vi "dI-dV(V)_two devices_MFLI_MF-MD_K3636B_PK_V4.0.vi"() -> ()   [LabVIEW 2016]
uses:
  <instrlib>/Keithley 2600 Series/Public/Configure/Source/Configure Source (Limit).vi
  <instrlib>/Keithley 2600 Series/Public/Configure/Source/Configure Source (Range).vi
  <instrlib>/Zurich Instruments LabOne/Public/Configure/ziSetValueDouble.vi
  <instrlib>/Zurich Instruments LabOne/Public/Configure/ziGetValueDemodSampleEx.vi
  <instrlib>/Zurich Instruments LabOne/Zurich Instruments LabOne.lvlib
  <instrlib>/Keithley 2600 Series/Keithley 2600 Series.lvlib
panel:
  in  "MFLI autorange":bool
  in  "MFLI autophase":bool=TRUE
  out "data 2":dbl[](array[numeric])=[4987.521, -0.0022013766920000004, 3.480726954118042e-11, 5.034309826469514e-06, 6.914010210132466e-06, -1.6999999999999718, -8.499999999999859e-08]
  in  "Tab Control":enum32{"Device 1", "Device 2"}(tab)
  out "dI/dV vs DC Bias (Device 1)":cluster{dbl, "Field Reading":dbl}[](graph)=[{0.0014399891434999999, "Field Reading"=3.539984741655203e-05}, {0.0015442875115, "Field Reading"=3.479350977367112e-05}, {0.0015470007610000002, "Field Reading"=3.023097158131358e-05}, {0.00154666596, "Field Reading"=2.8749503676306814e-05}, {0.0015427451470000002, "Field Reading"=3.1774133983659106e-05}, {0.001535730355, "Field Reading"=3.5727767936050286e-05}, {0.001534129679, "Field Reading"=3.5111822569235866e-05}, {0.0015285104130000002, "Field Reading"=2.941147033935653e-05}, {0.0015257152995, "Field Reading"=2.9865278120159806e-05}, {0.0015236269315000001, "Field Reading"=3.240454202938594e-05}, {0.0015206740594999998, "Field Reading"=3.325907996536474e-05}, {0.0015153374560000004, "Field Reading"=3.1387152081909155e-05}, {0.001509890312, "Field Reading"=2.996223500052808e-05}, {0.0015049572590000002, "Field Reading"=3.099093031549478e-05}, {0.0015046650365000002, "Field Reading"=3.2089661815348154e-05}, {0.0015006593160000004, "Field Reading"=3.401106812223111e-05}, {0.001496798368, "Field Reading"=3.072884553542488e-05}, {0.001492131612, "Field Reading"=2.9522459100156508e-05}, {0.001486837714, "Field Reading"=3.153606057559728e-05}, {0.001484281524, "Field Reading"=3.175161419362383e-05}, {0.0014819942635, "Field Reading"=3.1800258559693947e-05}, {0.001478613938, "Field Reading"=3.126830433448307e-05}, {0.001469819908, "Field Reading"=2.7391136145857723e-05}, {0.0014674311730000001, "Field Reading"=2.8763716237227997e-05}, {0.001466370573, "Field Reading"=3.1089573912688234e-05}, {0.001461121836, "Field Reading"=3.307180706002982e-05}, {0.001458794033, "Field Reading"=3.121787322651838e-05}, {0.0014529708325000002, "Field Reading"=2.8244891952200815e-05}, {0.0014474971195, "Field Reading"=2.825445502582387e-05}, {0.0014433356870000003, "Field Reading"=3.072241009524203e-05}, {0.001438264611, "Field Reading"=2.995842383800983e-05}, {0.001435399206, "Field Reading"=3.3231202804746765e-05}, {0.0014323585335, "Field Reading"=3.1872234223847094e-05}, {0.0014242775069999998, "Field Reading"=3.0354032499741767e-05}, {0.0014239959914999999, "Field Reading"=3.237759520768794e-05}, {0.0014193896074999998, "Field Reading"=3.0402839737892528e-05}, {0.0014128105435000002, "Field Reading"=2.9377356291311724e-05}, {0.0014078315605000002, "Field Reading"=2.7797475631119178e-05}, {0.0014048058534999997, "Field Reading"=3.220364336714182e-05}, {0.001402497608, "Field Reading"=2.965534195305068e-05}, {0.0013961798765, "Field Reading"=3.067447845354369e-05}, {0.001390925393, "Field Reading"=3.11703676364192e-05}, {0.0013872433314999998, "Field Reading"=2.9243257786824305e-05}, {0.0013821559399999999, "Field Reading"=2.7398973790428333e-05}, {0.001377423483, "Field Reading"=3.008617236104539e-05}, {0.0013727005385, "Field Reading"=2.8406131733354052e-05}, {0.0013678423729999998, "Field Reading"=3.104440370058421e-05}, {0.0013666582235, "Field Reading"=3.047636089229375e-05}, {0.0013646590885000001, "Field Reading"=3.0184765629058295e-05}, {0.0013589371445, "Field Reading"=3.0307666179171986e-05}, {0.0013560817375000002, "Field Reading"=2.9523004632232655e-05}, {0.0013515789905000001, "Field Reading"=3.082554161062039e-05}, {0.0013447046144999999, "Field Reading"=3.106728717375647e-05}, {0.0013385220485, "Field Reading"=2.974868707473485e-05}, {0.0013374483420000003, "Field Reading"=2.8651427002743325e-05}, {0.0013321132029999998, "Field Reading"=3.055303541114044e-05}, {0.0013274556029999997, "Field Reading"=3.0637799613688364e-05}, {0.001321575341, "Field Reading"=3.1304129713072345e-05}, {0.0013141655734999998, "Field Reading"=2.7826668858596676e-05}, {0.0013122313234999999, "Field Reading"=2.938837368452147e-05}, {0.001307794673, "Field Reading"=3.2897151730779044e-05}, {0.0013034739785, "Field Reading"=3.0675530645251095e-05}, {0.001297746598, "Field Reading"=3.097612663835991e-05}, {0.0012949037034999998, "Field Reading"=3.226733852363065e-05}, {0.0012919954510000001, "Field Reading"=2.905384119263297e-05}, {0.0012888060755, "Field Reading"=2.9760444377154905e-05}, {0.0012821942274999997, "Field Reading"=3.152958550570822e-05}, {0.00127900604, "Field Reading"=2.9754485932266634e-05}, {0.0012753080475000002, "Field Reading"=2.7941981758265642e-05}, {0.001271380758, "Field Reading"=2.897923489602027e-05}, {0.0012681222019999998, "Field Reading"=3.0145087015586976e-05}, {0.0012625594059999998, "Field Reading"=2.9888548610541235e-05}, {0.0012601185500000001, "Field Reading"=2.892551585933325e-05}, {0.0012563334949999999, "Field Reading"=2.914199842671685e-05}, {0.0012516522169999998, "Field Reading"=3.106836766844688e-05}, {0.0012466661809999997, "Field Reading"=2.931506336795828e-05}, {0.0012434836825, "Field Reading"=3.012840945054606e-05}, {0.001238093922, "Field Reading"=3.013433569745804e-05}, {0.001232953168, "Field Reading"=2.8832248492968933e-05}, {0.0012277401725000003, "Field Reading"=2.8988694843593325e-05}, {0.0012234111989999998, "Field Reading"=3.0242812296195605e-05}, {0.0012216526839999998, "Field Reading"=3.089554375166708e-05}, {0.0012165614215, "Field Reading"=2.8698972585958197e-05}, {0.0012121334570000001, "Field Reading"=2.8319095802121462e-05}, {0.0012098926105, "Field Reading"=2.763785246347619e-05}, {0.0012050341640000002, "Field Reading"=2.973094124014038e-05}, {0.0012014678839999998, "Field Reading"=3.119323554533092e-05}, {0.00119644038, "Field Reading"=2.898124104108434e-05}, {0.001191083737, "Field Reading"=2.820127031302108e-05}, {0.0011860875315, "Field Reading"=2.798966210613631e-05}, {0.001181310497, "Field Reading"=3.053637390193424e-05}, {0.0011761192575000003, "Field Reading"=2.81047730972618e-05}, {0.001171179016, "Field Reading"=2.9913610446049883e-05}, {0.001166600119, "Field Reading"=2.9097237815217114e-05}, {0.0011662118055, "Field Reading"=2.9262892022534514e-05}, {0.0011637166605, "Field Reading"=2.7160091515073227e-05}, {0.0011595062940000002, "Field Reading"=2.7876172605800874e-05}, {0.0011525607660000004, "Field Reading"=2.9328265579124486e-05}, {0.0011474100155, "Field Reading"=2.780060002119802e-05}, {0.0011431688820000001, "Field Reading"=2.869299201580142e-05}, {0.0011373234735, "Field Reading"=2.9999385402787912e-05}, {0.0011332899885000002, "Field Reading"=2.7787092135107974e-05}, {0.0011274989709999998, "Field Reading"=2.832686477947079e-05}, {0.001121785455, "Field Reading"=2.877980796483004e-05}, {0.00111626547, "Field Reading"=2.9505815517494233e-05}, {0.0011128954825, "Field Reading"=2.6724980409852468e-05}, {0.001108690413, "Field Reading"=2.949081340220257e-05}, {0.0011035870930000001, "Field Reading"=2.893692751618776e-05}, {0.0010992904555, "Field Reading"=2.8973874312015976e-05}, {0.0010952211570000002, "Field Reading"=2.7947861861950238e-05}, {0.0010945930425, "Field Reading"=2.679006764938657e-05}, {0.001090257549, "Field Reading"=2.941158012860888e-05}, {0.0010852873185000001, "Field Reading"=2.865060713681523e-05}, {0.0010813640165000002, "Field Reading"=2.847363898604231e-05}, {0.0010766837349999998, "Field Reading"=2.7137000104643942e-05}, {0.0010729132935, "Field Reading"=2.7304465600784156e-05}, {0.001065158915, "Field Reading"=2.9474555033440265e-05}, {0.0010584838075000003, "Field Reading"=2.8951717323060825e-05}, {0.001055930303, "Field Reading"=2.8197744534596472e-05}, {0.001051506708, "Field Reading"=2.813935590078248e-05}, {0.001048655317, "Field Reading"=2.7457099511248944e-05}, {0.0010452859699999998, "Field Reading"=2.8129650859824848e-05}, {0.0010392103565000001, "Field Reading"=2.8386664538660484e-05}, {0.0010361408315, "Field Reading"=2.9145292073684028e-05}, {0.0010294199855, "Field Reading"=2.69594894037016e-05}, {0.001023745664, "Field Reading"=2.8633350551353477e-05}, {0.0010203086779999998, "Field Reading"=2.849731787795889e-05}, {0.0010141151010000004, "Field Reading"=2.83146550303579e-05}, {0.001008619177, "Field Reading"=2.773198825459167e-05}, {0.001002912347, "Field Reading"=2.725891765436985e-05}, {0.0009962556867, "Field Reading"=2.872385890178788e-05}, {0.00099223266475, "Field Reading"=2.708421117774275e-05}, {0.0009906227914999997, "Field Reading"=2.8873027104615078e-05}, {0.0009858544061999998, "Field Reading"=2.823219667588614e-05}, {0.00098009373775, "Field Reading"=2.775224423256098e-05}, {0.0009751813368, "Field Reading"=2.7704772924742456e-05}, {0.0009701312228999998, "Field Reading"=2.873380694247318e-05}, {0.0009644217738, "Field Reading"=2.6861226192122225e-05}, {0.0009578559449999998, "Field Reading"=2.85256105088142e-05}, {0.0009539425876000001, "Field Reading"=2.7924498092117206e-05}, {0.0009513818346500001, "Field Reading"=2.6099498824452862e-05}, {0.0009462421892499999, "Field Reading"=2.709904571514122e-05}, {0.0009418883127499999, "Field Reading"=2.768778165159705e-05}, {0.00093742923265, "Field Reading"=2.744018195436568e-05}, {0.0009327565449000002, "Field Reading"=2.6443486426550465e-05}, {0.0009290616069500001, "Field Reading"=2.7514798871704233e-05}, {0.00092673901585, "Field Reading"=2.794358683356436e-05}, {0.0009203088168000001, "Field Reading"=2.770115760603011e-05}, {0.0009145794246999999, "Field Reading"=2.7636471710395534e-05}, {0.00090842506875, "Field Reading"=2.6764078766304754e-05}, {0.00090077597955, "Field Reading"=2.7150526980398903e-05}, {0.00089646212625, "Field Reading"=2.7520786364024458e-05}, {0.0008906256886000002, "Field Reading"=2.7831637446333116e-05}, {0.0008856995292, "Field Reading"=2.631326422089245e-05}, {0.0008836259033, "Field Reading"=2.8233537331017953e-05}, {0.0008791930340999999, "Field Reading"=2.706401776615399e-05}, {0.00087525207395, "Field Reading"=2.7520214395887868e-05}, {0.0008724134060500001, "Field Reading"=2.8272804485753116e-05}, {0.0008646784291999998, "Field Reading"=2.731466430586837e-05}, {0.0008590569936000001, "Field Reading"=2.644908415508535e-05}, {0.0008540370289, "Field Reading"=2.652451844467208e-05}, {0.0008494558809500001, "Field Reading"=2.653246513039182e-05}, {0.0008430573263999999, "Field Reading"=2.717732781056327e-05}, {0.0008384341093, "Field Reading"=2.6343442524410912e-05}, {0.0008339046709999999, "Field Reading"=2.7015478964114357e-05}, {0.0008288371037499999, "Field Reading"=2.683564270016631e-05}, {0.0008243482518, "Field Reading"=2.7061071714567523e-05}, {0.0008224905806500001, "Field Reading"=2.7833471132280706e-05}, {0.0008167230211, "Field Reading"=2.7130822144725484e-05}, {0.0008139826599, "Field Reading"=2.7002573082600767e-05}, {0.00081011256475, "Field Reading"=2.6699793633173424e-05}, {0.00080354357335, "Field Reading"=2.6601707234183626e-05}, {0.0007998235963500002, "Field Reading"=2.7518846084862328e-05}, {0.00079305690065, "Field Reading"=2.5933886336674594e-05}, {0.0007881982002, "Field Reading"=2.628432329552786e-05}, {0.0007849861712, "Field Reading"=2.731155419644831e-05}, {0.00077924129495, "Field Reading"=2.6498316239054298e-05}, {0.00077386634115, "Field Reading"=2.661237385473222e-05}, {0.000772586717, "Field Reading"=2.683367763980429e-05}, {0.00076715324385, "Field Reading"=2.7552914639933646e-05}, {0.00076283068005, "Field Reading"=2.529660873922404e-05}, {0.0007584143292500001, "Field Reading"=2.6813040060921684e-05}, {0.0007518176841999999, "Field Reading"=2.6098759138522866e-05}, {0.0007503320720500001, "Field Reading"=2.7584507574510233e-05}, {0.0007454194233999999, "Field Reading"=2.6381757940346435e-05}, {0.0007392297915499999, "Field Reading"=2.6664197485017493e-05}, {0.0007335713615, "Field Reading"=2.5833327337248065e-05}, {0.0007310102463, "Field Reading"=2.6845579698123368e-05}, {0.0007250234232999999, "Field Reading"=2.5419589094556693e-05}, {0.0007188638338, "Field Reading"=2.664214168588533e-05}, {0.0007165599543499999, "Field Reading"=2.5592852741351857e-05}, {0.0007119381531, "Field Reading"=2.6259267949927292e-05}, {0.0007098633958499999, "Field Reading"=2.673315141982664e-05}, {0.0007047486914500001, "Field Reading"=2.6457039708447496e-05}, {0.0007025036933500001, "Field Reading"=2.5257856553764385e-05}, {0.0006956025043, "Field Reading"=2.628501082062639e-05}, {0.0006888174652, "Field Reading"=2.6144779354954198e-05}, {0.00068248965275, "Field Reading"=2.59082571996256e-05}, {0.0006772642433000001, "Field Reading"=2.5689649875885376e-05}, {0.0006708514852, "Field Reading"=2.6521326635999304e-05}, {0.0006693603533000001, "Field Reading"=2.548743026040851e-05}, {0.00066562013705, "Field Reading"=2.5431203693357216e-05}, {0.0006597756623499999, "Field Reading"=2.500251770448019e-05}, {0.0006545812863499999, "Field Reading"=2.5962650488942607e-05}, {0.00064974467235, "Field Reading"=2.5816920621354972e-05}, {0.0006442822826, "Field Reading"=2.5159993064492232e-05}, {0.0006390915108499999, "Field Reading"=2.660956856843091e-05}, {0.0006341380824, "Field Reading"=2.4788097750258985e-05}, {0.00062805348185, "Field Reading"=2.5239440389139205e-05}, {0.00062110338895, "Field Reading"=2.4843288989688017e-05}, {0.0006170477987, "Field Reading"=2.5471157379008036e-05}, {0.00061183636825, "Field Reading"=2.5198329240766945e-05}, {0.00060867340895, "Field Reading"=2.5026640430883117e-05}, {0.0006043969231999999, "Field Reading"=2.4532829122884805e-05}, {0.00059734108645, "Field Reading"=2.548186660127621e-05}, {0.0005915697426, "Field Reading"=2.53532964278651e-05}, {0.0005844833989, "Field Reading"=2.423295748808172e-05}, {0.0005813260316, "Field Reading"=2.530045533051123e-05}, {0.0005753792359999999, "Field Reading"=2.460499357020733e-05}, {0.00056967967195, "Field Reading"=2.476774868624248e-05}, {0.0005661936702499998, "Field Reading"=2.509068143160599e-05}, {0.0005608593239499999, "Field Reading"=2.508099804473662e-05}, {0.0005529609736, "Field Reading"=2.434759142994004e-05}, {0.0005465511633000001, "Field Reading"=2.472033680947642e-05}, {0.0005420742435999999, "Field Reading"=2.5294665456280207e-05}, {0.0005380521151000001, "Field Reading"=2.4446332182633667e-05}, {0.00053460002175, "Field Reading"=2.5219944239969312e-05}, {0.0005282012281499999, "Field Reading"=2.4927595151619875e-05}, {0.0005243503773499999, "Field Reading"=2.429086406589632e-05}, {0.000520241094, "Field Reading"=2.447064522503621e-05}, {0.0005154410257000001, "Field Reading"=2.4998108009755677e-05}, {0.0005086838760999998, "Field Reading"=2.4879104926386617e-05}, {0.0005030509692, "Field Reading"=2.52088880671345e-05}, {0.00049863510835, "Field Reading"=2.4460419844711307e-05}, {0.00049550265335, "Field Reading"=2.4131581166292184e-05}, {0.0004905697873499999, "Field Reading"=2.494270174489369e-05}, {0.00048358716750000004, "Field Reading"=2.4212429855592305e-05}, {0.00047998159185, "Field Reading"=2.456164211241159e-05}, {0.00047376262365, "Field Reading"=2.4452567434274788e-05}, {0.00046960355054999987, "Field Reading"=2.412365841886655e-05}, {0.00046395107535, "Field Reading"=2.468534893656029e-05}, {0.00045919463465, "Field Reading"=2.4664106355610692e-05}, {0.0004560322024, "Field Reading"=2.4709306593844774e-05}, {0.00045091883165, "Field Reading"=2.5036193006732655e-05}, {0.00044793911940000004, "Field Reading"=2.4227487109089688e-05}, {0.00044306784715, "Field Reading"=2.517362154516144e-05}, {0.0004394137854, "Field Reading"=2.4822170605215546e-05}, {0.0004343439982, "Field Reading"=2.4826098311102026e-05}, {0.00043020854309999993, "Field Reading"=2.4365481177436e-05}, {0.00042386048834999995, "Field Reading"=2.4189633858249927e-05}, {0.0004200018422500001, "Field Reading"=2.493572935828982e-05}, {0.00041879972499999995, "Field Reading"=2.5612108271423455e-05}, {0.0004126587697999999, "Field Reading"=2.4877559496683757e-05}, {0.00040355976715, "Field Reading"=2.4722490914043894e-05}, {0.00039708264615, "Field Reading"=2.507577663272283e-05}, {0.0003926418904, "Field Reading"=2.4859213827902027e-05}, {0.00038827582905000003, "Field Reading"=2.484408253104443e-05}, {0.00038332477235000003, "Field Reading"=2.4704709168198052e-05}, {0.00037710729935000004, "Field Reading"=2.449886332521343e-05}, {0.00036955482050000005, "Field Reading"=2.492090369325475e-05}, {0.00036543200345000006, "Field Reading"=2.5169323793221225e-05}, {0.0003600878789, "Field Reading"=2.4800261123674807e-05}, {0.0003548235144, "Field Reading"=2.4379325397423533e-05}, {0.00035248225715, "Field Reading"=2.5072746136214913e-05}, {0.00034454190035000003, "Field Reading"=2.5456751026618948e-05}, {0.0003373547338, "Field Reading"=2.5193594542978225e-05}, {0.00033139157100000005, "Field Reading"=2.5051119772538443e-05}, {0.00032845802785000003, "Field Reading"=2.4595954455078518e-05}, {0.00031977012094999994, "Field Reading"=2.5555066907659082e-05}, {0.00031229189740000004, "Field Reading"=2.525033796639999e-05}, {0.0003070755153, "Field Reading"=2.4959636421672204e-05}, {0.00030173855935, "Field Reading"=2.511727230190406e-05}, {0.00029700412215000004, "Field Reading"=2.485646423766272e-05}, {0.00029108035300000004, "Field Reading"=2.5254110212854904e-05}, {0.00028656948975, "Field Reading"=2.522063844237432e-05}, {0.00028121404, "Field Reading"=2.556225551518139e-05}, {0.0002768915544, "Field Reading"=2.5348455473893375e-05}, {0.00027314623445, "Field Reading"=2.596928765567297e-05}, {0.0002686946441, "Field Reading"=2.5794692974694497e-05}, {0.00026405435680000003, "Field Reading"=2.543835530019002e-05}, {0.00025547767255, "Field Reading"=2.5967526298170223e-05}, {0.00025577685035000004, "Field Reading"=2.5919987667737076e-05}, {0.0002475684079, "Field Reading"=2.6727985706790567e-05}, {0.00024244191250000002, "Field Reading"=2.6286364593496668e-05}, {0.00023755152825, "Field Reading"=2.6064537241575083e-05}, {0.00023369517364999997, "Field Reading"=2.644985803858201e-05}, {0.00022849653985000003, "Field Reading"=2.6469041455970916e-05}, {0.00022485788605, "Field Reading"=2.6674888198321487e-05}, {0.00021704982410000002, "Field Reading"=2.6884455180053248e-05}, {0.00021395987409999996, "Field Reading"=2.6883046699655776e-05}, {0.00020615774949999998, "Field Reading"=2.691626478195444e-05}, {0.00019933952025000002, "Field Reading"=2.7295263506282656e-05}, {0.00019463775365, "Field Reading"=2.737091952442337e-05}, {0.0001917452195, "Field Reading"=2.750745359434406e-05}, {0.00018569049294999999, "Field Reading"=2.8296354710335358e-05}, {0.0001812998034, "Field Reading"=2.8517056990434556e-05}, {0.00017823559865000002, "Field Reading"=2.8593356237518392e-05}, {0.0001737937612, "Field Reading"=2.861871554641695e-05}, {0.0001700427832, "Field Reading"=2.882651694872817e-05}, {0.00016924993275000002, "Field Reading"=2.9231417800203077e-05}, {0.00016525125185, "Field Reading"=2.9408133529936847e-05}, {0.00016064549415, "Field Reading"=2.9491500714110673e-05}, {0.00015722823585, "Field Reading"=3.06834394085974e-05}, {0.00015247696070000002, "Field Reading"=3.1570866964132345e-05}, {0.00014844088830000003, "Field Reading"=3.0781559929643716e-05}, {0.00014316816515, "Field Reading"=3.1728014939431126e-05}, {0.00013987931785, "Field Reading"=3.2125458999320914e-05}, {0.00013671200479999999, "Field Reading"=3.284340832072761e-05}, {0.0001366118402, "Field Reading"=3.3356574795994144e-05}, {0.00013220151095, "Field Reading"=3.440093673855362e-05}, {0.00012683921535, "Field Reading"=3.527437392777797e-05}, {0.00012226255275, "Field Reading"=3.521770490817976e-05}, {0.00011886821990000002, "Field Reading"=3.7293066150943776e-05}, {0.00011505580454999999, "Field Reading"=3.7984175461221217e-05}, {0.00011490839619999998, "Field Reading"=3.876432629075614e-05}, {0.00011242408390000002, "Field Reading"=3.978183890147552e-05}, {0.00011095500830000001, "Field Reading"=4.088599194523828e-05}, {0.00010964993754999999, "Field Reading"=4.234633944029058e-05}, {0.00010712797994999999, "Field Reading"=4.323003495776657e-05}, {0.00010219273870000001, "Field Reading"=4.3184482483381195e-05}, {9.631986105499999e-05, "Field Reading"=4.5991318352294254e-05}, {9.527548263e-05, "Field Reading"=4.7847802385840867e-05}, {9.252191591499999e-05, "Field Reading"=4.989054521708996e-05}, {8.8617183645e-05, "Field Reading"=5.046410957067126e-05}, {8.7566451025e-05, "Field Reading"=5.246608919854773e-05}, {8.3063985815e-05, "Field Reading"=5.321509081606504e-05}, {8.1176531035e-05, "Field Reading"=5.4582323046123394e-05}, {7.907132144500001e-05, "Field Reading"=5.5596712751055124e-05}, {7.827213049e-05, "Field Reading"=5.375508176128449e-05}, {7.841774079000001e-05, "Field Reading"=5.41199224112345e-05}, {7.4509621425e-05, "Field Reading"=5.2990999011949546e-05}, {7.320589597999999e-05, "Field Reading"=4.9695563411219837e-05}, {6.864829185e-05, "Field Reading"=4.520530671515756e-05}, {6.768719516000001e-05, "Field Reading"=4.0779634591056634e-05}, {6.4593064545e-05, "Field Reading"=3.5474813084590765e-05}, {6.2432785315e-05, "Field Reading"=3.084529558773287e-05}, {5.670509802000001e-05, "Field Reading"=2.4482478477827943e-05}, {5.3037691230000004e-05, "Field Reading"=1.773821775920651e-05}, {3.9517599785e-05, "Field Reading"=1.1809336674850649e-05}, {2.3342955355e-05, "Field Reading"=6.418252148735044e-06}, {-2.3944236415e-05, "Field Reading"=1.2874313254256006e-06}, {-0.00044288596725000005, "Field Reading"=1.7829705228301125e-06}, {-0.0005051536444, "Field Reading"=7.727922995125912e-06}, {-0.0005184544644500001, "Field Reading"=1.2556664668411418e-05}, {-0.0005268976066, "Field Reading"=1.8327868347778772e-05}, {-0.0005357643552, "Field Reading"=2.5035434821338e-05}, {-0.00053897130225, "Field Reading"=3.005580738892413e-05}, {-0.0005437766682, "Field Reading"=3.5395922163059525e-05}, {-0.00054553804945, "Field Reading"=4.150184448391502e-05}, {-0.0005511706686500001, "Field Reading"=4.6362694015758234e-05}, {-0.0005559163023499999, "Field Reading"=5.0130423425832106e-05}, {-0.0005543881889499999, "Field Reading"=5.335741502524605e-05}, {-0.0005592604063, "Field Reading"=5.411570066512388e-05}, {-0.0005605982064999999, "Field Reading"=5.465121419090429e-05}, {-0.0005629030597, "Field Reading"=5.475473056047824e-05}, {-0.0005643864397499999, "Field Reading"=5.501166190948225e-05}, {-0.0005697240176, "Field Reading"=5.31400833500483e-05}, {-0.0005718998929, "Field Reading"=5.319476368452034e-05}, {-0.0005761703489, "Field Reading"=5.0393322614515415e-05}, {-0.0005774828608, "Field Reading"=5.0117210546142615e-05}, {-0.0005792511608, "Field Reading"=4.763450052536487e-05}, {-0.00058427729175, "Field Reading"=4.6222596298617735e-05}, {-0.0005839630306500001, "Field Reading"=4.380763636273433e-05}, {-0.00058690824465, "Field Reading"=4.341709663323534e-05}, {-0.00058665562145, "Field Reading"=4.257979811006354e-05}, {-0.00059081148145, "Field Reading"=3.9733022729478504e-05}, {-0.0005917890384000001, "Field Reading"=3.922882008869421e-05}, {-0.0005928376371999999, "Field Reading"=3.872769287644023e-05}, {-0.0005963710346499999, "Field Reading"=3.786839615999292e-05}, {-0.00060304377145, "Field Reading"=3.614498242064283e-05}, {-0.00060705747125, "Field Reading"=3.5275522377934295e-05}, {-0.0006140201557499999, "Field Reading"=3.473781066261673e-05}, {-0.0006186047409, "Field Reading"=3.417365953948509e-05}, {-0.0006230151480999999, "Field Reading"=3.3079225624050956e-05}, {-0.0006267799413000001, "Field Reading"=3.251474967299545e-05}, {-0.00062886941835, "Field Reading"=3.2595210913017203e-05}, {-0.0006354146897, "Field Reading"=3.1488792156517215e-05}, {-0.0006380160867000001, "Field Reading"=3.120214389597704e-05}, {-0.00064386830235, "Field Reading"=3.125684953560282e-05}, {-0.0006480523066999999, "Field Reading"=3.0277268568468644e-05}, {-0.00064896883845, "Field Reading"=2.9768651422877856e-05}, {-0.00065340680835, "Field Reading"=2.960934130033152e-05}, {-0.00065811164405, "Field Reading"=2.9778240274563194e-05}, {-0.0006635885125500002, "Field Reading"=2.9376542680395736e-05}, {-0.00066648116515, "Field Reading"=2.852598488267133e-05}, {-0.0006695975924, "Field Reading"=2.7962131958752747e-05}, {-0.0006771186086500001, "Field Reading"=2.792167139815216e-05}, {-0.00067967447245, "Field Reading"=2.8593051848648095e-05}, {-0.0006853313692000001, "Field Reading"=2.827992652732514e-05}, {-0.00068965257765, "Field Reading"=2.733016829877469e-05}, {-0.00069658048195, "Field Reading"=2.718001106596477e-05}, {-0.00070006927375, "Field Reading"=2.697314805126955e-05}, {-0.0007063067703, "Field Reading"=2.7223623241350286e-05}, {-0.0007104617050500001, "Field Reading"=2.7221131662322604e-05}, {-0.0007158454615000001, "Field Reading"=2.6470268262583008e-05}, {-0.0007208107891, "Field Reading"=2.6360429428319376e-05}, {-0.00072542920115, "Field Reading"=2.6359508605806887e-05}, {-0.00073385787325, "Field Reading"=2.6465138066782306e-05}, {-0.0007344708868000001, "Field Reading"=2.5871440569675743e-05}, {-0.0007403752824, "Field Reading"=2.6927353113657345e-05}, {-0.0007431207725999999, "Field Reading"=2.5848786429398566e-05}, {-0.0007452998807500001, "Field Reading"=2.6119694708101804e-05}, {-0.0007487942998500001, "Field Reading"=2.636072535607038e-05}, {-0.0007553057972000001, "Field Reading"=2.6220748174400285e-05}, {-0.0007591562609500001, "Field Reading"=2.5886324889822564e-05}, {-0.0007657129732500001, "Field Reading"=2.553410085362131e-05}, {-0.0007685236647999999, "Field Reading"=2.5299635240635863e-05}, {-0.00077290691525, "Field Reading"=2.55529616681101e-05}, {-0.0007775658146, "Field Reading"=2.5593459123952253e-05}, {-0.00078298779045, "Field Reading"=2.5766911715028896e-05}, {-0.0007868718035000001, "Field Reading"=2.5329800845548382e-05}, {-0.00079214363745, "Field Reading"=2.5111997926056203e-05}, {-0.00079630611485, "Field Reading"=2.5219866414641062e-05}, {-0.0008009303386, "Field Reading"=2.576886341774044e-05}, {-0.0008081203436000001, "Field Reading"=2.5191674409460277e-05}, {-0.0008128989841, "Field Reading"=2.4659895923638357e-05}, {-0.00081992365215, "Field Reading"=2.557847433769245e-05}, {-0.0008227442695, "Field Reading"=2.491401355296153e-05}, {-0.0008269649726, "Field Reading"=2.494049970344901e-05}, {-0.0008320200444000001, "Field Reading"=2.498865870175516e-05}, {-0.0008362681799499999, "Field Reading"=2.507156110645498e-05}, {-0.00084043577685, "Field Reading"=2.4859819723508128e-05}, {-0.0008482895495, "Field Reading"=2.4756956203228876e-05}, {-0.0008519631337, "Field Reading"=2.514257946106073e-05}, {-0.00085482501865, "Field Reading"=2.5190629511597944e-05}, {-0.00086115240905, "Field Reading"=2.4968169535876815e-05}, {-0.0008669621674000001, "Field Reading"=2.46774175944596e-05}, {-0.0008739308819, "Field Reading"=2.4956204388644077e-05}, {-0.00087753713925, "Field Reading"=2.501595182353837e-05}, {-0.0008833726753999999, "Field Reading"=2.4753643027387e-05}, {-0.0008833791037499998, "Field Reading"=2.4572507911983235e-05}, {-0.0008900118714, "Field Reading"=2.452449557800081e-05}, {-0.0008975926323500002, "Field Reading"=2.5742257691681753e-05}, {-0.0009049993725499999, "Field Reading"=2.483570784067544e-05}, {-0.0009106274022499999, "Field Reading"=2.4632699872762128e-05}, {-0.0009144832965, "Field Reading"=2.500623968887879e-05}, {-0.0009195275330000001, "Field Reading"=2.4533211575573895e-05}, {-0.0009253394478499998, "Field Reading"=2.46566289914237e-05}, {-0.0009295518563999999, "Field Reading"=2.4711007529370937e-05}, {-0.0009339636874499998, "Field Reading"=2.494095987800124e-05}, {-0.0009419215269, "Field Reading"=2.488276682153817e-05}, {-0.0009440282936000001, "Field Reading"=2.5362278074920992e-05}, {-0.0009520676295000001, "Field Reading"=2.4875495822276945e-05}, {-0.0009562295733499999, "Field Reading"=2.471985815352984e-05}, {-0.00096403001325, "Field Reading"=2.501400012487715e-05}, {-0.0009668210693999998, "Field Reading"=2.504545001027246e-05}, {-0.0009700857615000001, "Field Reading"=2.4825614172064623e-05}, {-0.0009741633754, "Field Reading"=2.508908994201125e-05}, {-0.0009786747900500002, "Field Reading"=2.547992134200255e-05}, {-0.0009831387377500001, "Field Reading"=2.4987278578304335e-05}, {-0.00098489078335, "Field Reading"=2.4799577546204462e-05}, {-0.00099149049345, "Field Reading"=2.517378273657648e-05}, {-0.0010008897577999999, "Field Reading"=2.501285906441021e-05}, {-0.0010047693850000002, "Field Reading"=2.517146386711981e-05}, {-0.001010887702, "Field Reading"=2.474528686486035e-05}, {-0.0010154381795, "Field Reading"=2.517950175218433e-05}, {-0.0010194920305, "Field Reading"=2.4943020751004832e-05}, {-0.001025390771, "Field Reading"=2.5059853035305155e-05}, {-0.0010319175369999998, "Field Reading"=2.5111712727938145e-05}, {-0.0010339942155000001, "Field Reading"=2.4965884900478457e-05}, {-0.0010387866259999998, "Field Reading"=2.4624146165130197e-05}, {-0.0010432882684999999, "Field Reading"=2.4974885798460943e-05}, {-0.001050285043, "Field Reading"=2.549970160202571e-05}, {-0.0010532131215, "Field Reading"=2.509936185921828e-05}, {-0.0010605935165, "Field Reading"=2.4679251006447366e-05}, {-0.0010649837745, "Field Reading"=2.534172622465245e-05}, {-0.0010699723350000002, "Field Reading"=2.5117530228594704e-05}, {-0.0010740878005, "Field Reading"=2.550911754774814e-05}, {-0.0010803877715, "Field Reading"=2.5590996285863874e-05}, {-0.0010843786035, "Field Reading"=2.532765980863689e-05}, {-0.0010869649905000003, "Field Reading"=2.504883136678769e-05}, {-0.0010908974514999999, "Field Reading"=2.5356105465320954e-05}, {-0.0010965432235000001, "Field Reading"=2.619328160076385e-05}, {-0.0011007961549999998, "Field Reading"=2.5554603625258115e-05}, {-0.0011068035015, "Field Reading"=2.486060925242396e-05}, {-0.0011102547485, "Field Reading"=2.5991799787265172e-05}, {-0.001114113474, "Field Reading"=2.5382768369364457e-05}, {-0.001120774231, "Field Reading"=2.560148212416169e-05}, {-0.0011256925015, "Field Reading"=2.535548059743797e-05}, {-0.0011314602925, "Field Reading"=2.4739011324466265e-05}, {-0.001133669728, "Field Reading"=2.4926499499317303e-05}, {-0.0011401122615000002, "Field Reading"=2.6136534239552487e-05}, {-0.0011450076414999998, "Field Reading"=2.5417209022334496e-05}, {-0.0011529607145000001, "Field Reading"=2.5698245491377132e-05}, {-0.0011577730315, "Field Reading"=2.6174948723676456e-05}, {-0.0011613708525, "Field Reading"=2.659495330024166e-05}, {-0.0011653017159999998, "Field Reading"=2.636519742423141e-05}, {-0.0011721344295000003, "Field Reading"=2.570186047778655e-05}, {-0.0011761560885000001, "Field Reading"=2.580018779418553e-05}, {-0.0011814869265000002, "Field Reading"=2.679967128975373e-05}, {-0.0011864733475, "Field Reading"=2.6239134735091276e-05}, {-0.0011893287184999999, "Field Reading"=2.5374579332499126e-05}, {-0.0011953142824999998, "Field Reading"=2.5780689417062888e-05}, {-0.0011998791505, "Field Reading"=2.6470977603648504e-05}, {-0.0012066721364999999, "Field Reading"=2.664068368641496e-05}, {-0.0012114344315000002, "Field Reading"=2.632872486761017e-05}, {-0.0012160587375, "Field Reading"=2.5944407033586477e-05}, {-0.0012206377089999999, "Field Reading"=2.6334788208618243e-05}, {-0.0012236480440000002, "Field Reading"=2.670412347473009e-05}, {-0.0012285901605, "Field Reading"=2.6385921389739756e-05}, {-0.0012339220824999998, "Field Reading"=2.6999631404588567e-05}, {-0.0012376608755, "Field Reading"=2.6434169175038227e-05}, {-0.0012383639600000002, "Field Reading"=2.7166475988494615e-05}, {-0.001244508114, "Field Reading"=2.7006307012055734e-05}, {-0.0012503813314999998, "Field Reading"=2.6804753979359723e-05}, {-0.0012582029339999999, "Field Reading"=2.7125886090709387e-05}, {-0.0012611768514999998, "Field Reading"=2.6236926946293805e-05}, {-0.0012639195255000001, "Field Reading"=2.6782100715955357e-05}, {-0.0012664462864999998, "Field Reading"=2.6554221045846453e-05}, {-0.0012745661625000002, "Field Reading"=2.6738797232680578e-05}, {-0.0012795817480000002, "Field Reading"=2.612651037782988e-05}, {-0.001282848078, "Field Reading"=2.6570038951477157e-05}, {-0.0012915996034999998, "Field Reading"=2.6500769220546404e-05}, {-0.0012962128675, "Field Reading"=2.6356774643710844e-05}, {-0.0013026879300000003, "Field Reading"=2.6794012485918364e-05}, {-0.001306773918, "Field Reading"=2.7001691426995927e-05}, {-0.0013085944285, "Field Reading"=2.6839401737944833e-05}, {-0.0013154063285, "Field Reading"=2.75133916908824e-05}, {-0.0013198725589999996, "Field Reading"=2.6462978869963258e-05}, {-0.0013259697260000001, "Field Reading"=2.7091350944690248e-05}, {-0.0013300431595, "Field Reading"=2.684988080475616e-05}, {-0.0013364990009999997, "Field Reading"=2.6864969015282564e-05}, {-0.001340103434, "Field Reading"=2.7074621441558483e-05}, {-0.0013446258885, "Field Reading"=2.658828009406131e-05}, {-0.0013491423099999999, "Field Reading"=2.6963634968708878e-05}, {-0.0013542443670000002, "Field Reading"=2.691242477475801e-05}, {-0.0013551154554999997, "Field Reading"=2.7408320729240955e-05}, {-0.0013603372705, "Field Reading"=2.6575551393078534e-05}, {-0.0013646557795, "Field Reading"=2.7190974281437918e-05}, {-0.0013668146055000004, "Field Reading"=2.7091075111983577e-05}, {-0.001374753727, "Field Reading"=2.697325299903679e-05}, {-0.0013790293659999998, "Field Reading"=2.6961363555538916e-05}, {-0.00138246604, "Field Reading"=2.7520779720375435e-05}, {-0.0013878468099999999, "Field Reading"=2.718517663643333e-05}, {-0.0013928858559999998, "Field Reading"=2.7704228552271802e-05}, {-0.0014003405395000001, "Field Reading"=2.7411265301839192e-05}, {-0.0014052482485, "Field Reading"=2.670572063970964e-05}, {-0.0014094181559999998, "Field Reading"=2.726189036114562e-05}, {-0.0014162599145, "Field Reading"=2.681430077596952e-05}, {-0.0014206207965000001, "Field Reading"=2.7064647645767718e-05}, {-0.001422804084, "Field Reading"=2.8156356118263624e-05}, {-0.0014294806425000002, "Field Reading"=2.816675161874044e-05}, {-0.0014314233145, "Field Reading"=2.836763394568079e-05}, {-0.0014342185515, "Field Reading"=2.7308793127739642e-05}, {-0.001438674201, "Field Reading"=2.7657009178311895e-05}, {-0.0014409701235000001, "Field Reading"=2.7488171670496874e-05}, {-0.0014457268345, "Field Reading"=2.7798227130753798e-05}, {-0.0014498154880000001, "Field Reading"=2.8672170248405528e-05}, {-0.0014527951515000003, "Field Reading"=2.814285356967082e-05}, {-0.001459003039, "Field Reading"=2.82471579598307e-05}, {-0.0014630158200000002, "Field Reading"=2.8591425967924597e-05}, {-0.0014650744875, "Field Reading"=2.8631034080160183e-05}, {-0.0014712758715, "Field Reading"=2.668663665944264e-05}, {-0.0014757668640000001, "Field Reading"=2.8148492175449524e-05}, {-0.001482266591, "Field Reading"=2.763950928937077e-05}, {-0.0014872015745000002, "Field Reading"=2.8529012683654844e-05}, {-0.0014917270425, "Field Reading"=2.7165504576848428e-05}, {-0.0014975122574999997, "Field Reading"=2.9116578377773362e-05}, {-0.0015011177470000002, "Field Reading"=2.9099655059723038e-05}, {-0.0015038803205000002, "Field Reading"=2.8669345250550533e-05}, {-0.0015074313985, "Field Reading"=2.818280079714946e-05}, {-0.0015148559224999998, "Field Reading"=2.8215570568220332e-05}, {-0.001518905766, "Field Reading"=2.8610697108516978e-05}, {-0.0015222922020000002, "Field Reading"=2.9179363255422852e-05}, {-0.0015271702825, "Field Reading"=2.8297513239277402e-05}, {-0.0015295628110000002, "Field Reading"=2.6834126964094553e-05}, {-0.0015345809465, "Field Reading"=2.792914219067848e-05}, {-0.0015406848935000002, "Field Reading"=2.829254332544149e-05}, {-0.0015452536425, "Field Reading"=2.7468626467104844e-05}, {-0.0015502011235000001, "Field Reading"=2.8621735203641882e-05}, {-0.0015551437465, "Field Reading"=2.761130630469376e-05}, {-0.0015605372085, "Field Reading"=2.6936326850914844e-05}, {-0.00156492463, "Field Reading"=2.827693033016408e-05}, {-0.0015669900035, "Field Reading"=2.8411256496876676e-05}, {-0.001571965995, "Field Reading"=2.7943121786343522e-05}, {-0.0015753530605, "Field Reading"=2.8376384388796066e-05}, {-0.0015807512605, "Field Reading"=2.978102067631948e-05}, {-0.0015864854214999997, "Field Reading"=3.004064400789514e-05}, {-0.001591627528, "Field Reading"=2.8055249135705818e-05}, {-0.0015950191769999998, "Field Reading"=2.949038938594226e-05}, {-0.001598778914, "Field Reading"=2.9143754000256578e-05}, {-0.0016050448364999998, "Field Reading"=2.8098754487818475e-05}, {-0.001609540912, "Field Reading"=2.8442217210198144e-05}, {-0.0016140246455, "Field Reading"=2.985325361373035e-05}, {-0.0016178020025, "Field Reading"=2.8824802231216225e-05}, {-0.0016212227885, "Field Reading"=2.9469524633747556e-05}, {-0.0016286767495, "Field Reading"=2.9330753129539258e-05}, {-0.0016321227720000001, "Field Reading"=2.863090278005049e-05}, {-0.0016345999689999998, "Field Reading"=2.945281627501967e-05}, {-0.0016406766190000001, "Field Reading"=3.0509889915088457e-05}, {-0.0016433718110000003, "Field Reading"=2.8234805007257297e-05}, {-0.0016475666914999999, "Field Reading"=3.0100850627959698e-05}, {-0.0016489186579999998, "Field Reading"=2.9164854213138128e-05}, {-0.0016580827585, "Field Reading"=2.820079826409188e-05}, {-0.0016634588009999999, "Field Reading"=2.948371397680206e-05}, {-0.001666819524, "Field Reading"=3.158853041941357e-05}, {-0.0016682677344999996, "Field Reading"=2.9247798446691426e-05}, {-0.0016724487044999996, "Field Reading"=2.820867278535577e-05}, {-0.001675465457, "Field Reading"=2.9148426410644136e-05}, {-0.0016796926040000004, "Field Reading"=3.063202582139158e-05}, {-0.0016869314475000002, "Field Reading"=3.084701188943617e-05}, {-0.0016899639645000003, "Field Reading"=3.0370369902881822e-05}, {-0.0016937376340000001, "Field Reading"=2.7594955047741704e-05}, {-0.0016975268330000001, "Field Reading"=2.9553103747146036e-05}, {-0.0017007798195, "Field Reading"=3.098220513643231e-05}, {-0.0017058537240000002, "Field Reading"=3.148168938244963e-05}, {-0.0017080639914999998, "Field Reading"=2.9579034160154674e-05}, {-0.0017110607904999998, "Field Reading"=2.7611498995410022e-05}, {-0.00171618452, "Field Reading"=3.0474417966750653e-05}, {-0.0017202808825, "Field Reading"=3.070057693750096e-05}, {-0.001727383138, "Field Reading"=3.162016826431228e-05}, {-0.0017310668390000002, "Field Reading"=2.9615498667636423e-05}, {-0.0017346550049999999, "Field Reading"=2.7453062758722423e-05}, {-0.0017379636470000002, "Field Reading"=3.043968244331558e-05}, {-0.001743127447, "Field Reading"=3.17359438510126e-05}, {-0.0017448500155000002, "Field Reading"=2.839198714788124e-05}, {-0.0017493435330000005, "Field Reading"=2.9537518085808404e-05}, {-0.001755053409, "Field Reading"=3.0267484755413558e-05}, {-0.00176169259, "Field Reading"=2.898267506640183e-05}, {-0.001762598, "Field Reading"=3.0300716833725148e-05}, {-0.0017671871915000002, "Field Reading"=3.080667331394037e-05}, {-0.0017705653674999998, "Field Reading"=3.0361398500792185e-05}, {-0.0017746671585000002, "Field Reading"=3.1106312903425585e-05}, {-0.0017783549920000002, "Field Reading"=2.9862151905111414e-05}, {-0.0017815493589999998, "Field Reading"=2.8501485801207906e-05}, {-0.001785276159, "Field Reading"=3.076140660046423e-05}, {-0.0017922079725, "Field Reading"=2.9058295998685708e-05}, {-0.0017961523975, "Field Reading"=2.8734206677692602e-05}, {-0.001799212137, "Field Reading"=3.137923256237406e-05}, {-0.0018059357504999999, "Field Reading"=3.179509940643667e-05}, {-0.0018087371615, "Field Reading"=3.228147459514946e-05}, {-0.0018160808960000004, "Field Reading"=3.293210062424598e-05}, {-0.001820149226, "Field Reading"=2.9163517417526188e-05}, {-0.0018234938499999999, "Field Reading"=3.1017183743855944e-05}, {-0.0018273520249999999, "Field Reading"=3.221606893453561e-05}, {-0.0018319088200000003, "Field Reading"=3.192150001949322e-05}, {-0.0018365081444999998, "Field Reading"=2.9959217951422412e-05}, {-0.0018389348775000001, "Field Reading"=2.789130975261861e-05}, {-0.0018452034285000001, "Field Reading"=3.17080422471979e-05}, {-0.0018500183390000005, "Field Reading"=3.2394673320763635e-05}, {-0.0018521909855, "Field Reading"=2.965997929508729e-05}, {-0.0018548242490000002, "Field Reading"=3.097145110133598e-05}, {-0.001858377908, "Field Reading"=3.0337147697741198e-05}, {-0.0018604670740000003, "Field Reading"=3.1532452120555806e-05}, {-0.0018638291629999998, "Field Reading"=3.270858332747162e-05}, {-0.0018671888555, "Field Reading"=3.0894156475968046e-05}, {-0.0018717320815, "Field Reading"=2.845308959992079e-05}, {-0.0018754390465, "Field Reading"=3.060980262409263e-05}, {-0.00187866943, "Field Reading"=3.2072999511849786e-05}, {-0.0018851805094999997, "Field Reading"=3.2173443940677715e-05}, {-0.001889215759, "Field Reading"=2.7966094150345777e-05}, {-0.0018937420315000002, "Field Reading"=3.0311161349639648e-05}, {-0.001897686686, "Field Reading"=3.274133195580933e-05}, {-0.001903061709, "Field Reading"=3.4094299280965945e-05}, {-0.0019071081000000003, "Field Reading"=3.082707587247123e-05}, {-0.001909890899, "Field Reading"=2.9702084757446434e-05}, {-0.0019168490989999998, "Field Reading"=2.976508458726319e-05}, {-0.001920534376, "Field Reading"=3.2748509436225333e-05}, {-0.001924188862, "Field Reading"=3.094510845635821e-05}, {-0.0019281178400000001, "Field Reading"=2.9363437972452403e-05}, {-0.001935024801, "Field Reading"=2.965602205230533e-05}, {-0.0019368541310000001, "Field Reading"=3.349567018076371e-05}, {-0.0019395661065, "Field Reading"=3.11382374433274e-05}, {-0.0019443560055, "Field Reading"=3.272398904929557e-05}, {-0.0019478042074999996, "Field Reading"=2.9959093799175477e-05}, {-0.0019505890269999999, "Field Reading"=3.21476349140092e-05}, {-0.001955327842, "Field Reading"=3.481998753888036e-05}, {-0.001960148591, "Field Reading"=3.2242893449899114e-05}, {-0.0019617751235, "Field Reading"=2.8580219684115152e-05}, {-0.0019670099799999996, "Field Reading"=3.0965338889550495e-05}, {-0.001969988556, "Field Reading"=3.32122447642128e-05}, {-0.0019757059180000006, "Field Reading"=3.253687631425346e-05}, {-0.0019789746340000006, "Field Reading"=2.742705969097034e-05}, {-0.0019831723155000003, "Field Reading"=3.196348596581089e-05}, {-0.0019871198235000007, "Field Reading"=2.900741316885134e-05}, {-0.0019899086759999998, "Field Reading"=3.543967510024724e-05}, {-0.0019937853094999995, "Field Reading"=3.032039195721649e-05}, {-0.001997198822, "Field Reading"=3.124126865424502e-05}, {-0.002004981853, "Field Reading"=2.8959096894867582e-05}, {-0.0020066316215, "Field Reading"=2.738232973306536e-05}, {-0.0020110788365, "Field Reading"=3.162264271194698e-05}]
  out "DC Voltage (V)":dbl=-0.0020110788365
  out "dI (A)":dbl=8.848779425879616e-11
  out "dV (V)":dbl=2.798241597479316e-06
  out "dI/dV (ohm)":dbl=3.162264271194698e-05
  out "Vset (V)":dbl=-1.6999999999999718
  in  "Nanovoltmeter 2182A VISA (Device1)":refnum<visa-resource-name>="GPIB0::4::INSTR"
  in  "MFLI Device 1 Address\n(connected to Channel A of K2635B)":string="DEV4382"
  in  "File Name Device 1":string="005_MA2479_[Dev110]_40uV_50pA_17.7777Hz_4thorder_300ms_2T_measureX_float_20xaverage"
  in  "From 1":dbl[](array[numeric])=[1.645, 0.5, 0.025, -0.035, -0.54] min=-3000.0 max=3000.0 format="%.2e"
  in  "To 1":dbl[](array[numeric])=[0.5, 0.025, -0.035, -0.54, -1.65] min=-3000.0 max=3000.0 format="%.2e"
  in  "Step 1":dbl[](array[numeric])=[0.005, 0.002, 0.001, 0.002, 0.005] min=-3000.0 max=3000.0 format="%.1e"
  in  "Resistance used for DC (Device 1) (ohm)":dbl=40000000.0 format="%#_13g"
  in  "DC Voltage averaging (Device 1)":dbl=20.0 format="%#_13g"
  in  "MFLI Averaging (Device1)":dbl=20.0 format="%#_13g"
  in  "MFLI Device 1 Delay (s)":dbl=4.0
  in  "MFLI Device 2 Address\n(connected to Channel B of K2635B)":string="DEV4496"
  in  "Resistance used for DC (ohm) 2":dbl=20000000.0 format="%#_13g"
  in  "Nanovoltmeter 2182a VISA (Device 2)":refnum<visa-resource-name>="GPIB0::7::INSTR"
  in  "File Name Device 2":string="006_MA2479_[Dev90]_40uV_33pA_7.919Hz_4thorder_300ms_2T_measureX_float_20xaverage"
  in  "MFLI Device 2 Delay (s)":dbl=4.0
  in  "From 3":dbl[](array[numeric])=[1.65, 0.5, 0.025, -0.035, -0.54] min=-3000.0 max=3000.0 format="%.2e"
  in  "To 3":dbl[](array[numeric])=[0.5, 0.025, -0.035, -0.54, 1.65] min=-3000.0 max=3000.0 format="%.2e"
  in  "Step 3":dbl[](array[numeric])=[0.005, 0.002, 0.001, 0.002, 0.005] min=-3000.0 max=3000.0 format="%.1e"
  out "dI/dV vs DC Bias (Device 2)":cluster{dbl, "Field Reading":dbl}[](graph)=[{0.0016536990575000004, "Field Reading"=1.0549538115165888e-05}, {0.001778714152, "Field Reading"=1.2441234786608795e-05}, {0.0017803415199999998, "Field Reading"=2.288258346714741e-05}, {0.0017755957270000002, "Field Reading"=1.318154414138772e-05}, {0.0017698667430000002, "Field Reading"=6.944765527644103e-06}, {0.0017656221274999998, "Field Reading"=1.2547089254133368e-05}, {0.0017618064770000004, "Field Reading"=8.29737778524207e-06}, {0.0017527998860000006, "Field Reading"=1.1494966792116706e-05}, {0.0017486110414999998, "Field Reading"=1.0588496845450188e-05}, {0.0017437714000000004, "Field Reading"=1.1963581383580064e-05}, {0.0017407059809999997, "Field Reading"=5.731216326454031e-06}, {0.0017423811614999999, "Field Reading"=5.30625093465625e-06}, {0.0017370860829999998, "Field Reading"=1.128100400443151e-05}, {0.0017338522185, "Field Reading"=2.123556094372534e-05}, {0.0017289355484999998, "Field Reading"=1.117670770827346e-05}, {0.0017188669980000002, "Field Reading"=1.0835120440598476e-05}, {0.0017189288765000002, "Field Reading"=2.0192283145985024e-05}, {0.0017122291565000002, "Field Reading"=2.4785742477983657e-05}, {0.0017076021445, "Field Reading"=1.0589077020565965e-05}, {0.0017052432175, "Field Reading"=1.3759186431392488e-05}, {0.0017045775195000002, "Field Reading"=1.537687077784978e-05}, {0.0016996537305, "Field Reading"=1.1320197025124775e-05}, {0.0016953896885, "Field Reading"=4.111009127394301e-06}, {0.001693602352, "Field Reading"=7.2063798052163e-06}, {0.0016863126914999998, "Field Reading"=7.631719043699821e-06}, {0.0016810597275000003, "Field Reading"=1.242338892269991e-05}, {0.001677800643, "Field Reading"=1.3726170510015826e-05}, {0.0016768591975, "Field Reading"=1.0512885770990247e-05}, {0.0016675404135000002, "Field Reading"=4.75578215245112e-06}, {0.0016654858590000002, "Field Reading"=2.027029645969641e-05}, {0.0016586733520000002, "Field Reading"=1.281946079436041e-05}, {0.0016534433870000003, "Field Reading"=6.055607337868207e-06}, {0.0016497589909999998, "Field Reading"=1.3221236417835137e-05}, {0.001642726164, "Field Reading"=8.223559087892218e-06}, {0.001632876745, "Field Reading"=1.590634888399578e-05}, {0.0016237432070000002, "Field Reading"=9.173376660503408e-06}, {0.0016184162055, "Field Reading"=1.6312838752629565e-05}, {0.001618065896, "Field Reading"=2.3731068197859222e-05}, {0.001618770715, "Field Reading"=1.0331543245369263e-05}, {0.0016073995474999998, "Field Reading"=6.470124896934937e-06}, {0.0015978612295, "Field Reading"=1.600525933976539e-05}, {0.0015944400540000001, "Field Reading"=1.7397689972344422e-05}, {0.0015942704750000001, "Field Reading"=1.2432826943314632e-05}, {0.0015882790550000002, "Field Reading"=9.114399852548662e-06}, {0.0015826422325, "Field Reading"=9.258860509987068e-06}, {0.0015787430519999999, "Field Reading"=1.8612913508766953e-05}, {0.001574898086, "Field Reading"=1.3182472661864731e-05}, {0.0015700212479999999, "Field Reading"=1.7030521500463586e-05}, {0.0015719165115, "Field Reading"=1.3417541074045366e-05}, {0.0015680138215, "Field Reading"=9.850868553296031e-06}, {0.00156138302, "Field Reading"=1.2254888938026482e-05}, {0.0015595287044999997, "Field Reading"=2.0389817245679517e-05}, {0.0015526102765, "Field Reading"=7.176125737368203e-06}, {0.0015470934585, "Field Reading"=1.474392740423153e-05}, {0.0015406487560000002, "Field Reading"=6.692190816914176e-06}, {0.0015367547195000001, "Field Reading"=1.5447400080198977e-05}, {0.001535941625, "Field Reading"=6.532333325868927e-06}, {0.0015307425095000002, "Field Reading"=1.7413230844513688e-05}, {0.0015260549489999999, "Field Reading"=1.0434230642215218e-05}, {0.0015176100955, "Field Reading"=1.2101733376211772e-05}, {0.001511127055, "Field Reading"=1.0178996127798104e-05}, {0.001507063141, "Field Reading"=1.4738737572511442e-05}, {0.0015027795215, "Field Reading"=8.262259757536864e-06}, {0.0014955986639999998, "Field Reading"=1.6465762643777065e-05}, {0.001489394298, "Field Reading"=1.426412095304383e-05}, {0.0014849224090000002, "Field Reading"=4.5222377370536295e-06}, {0.0014789590254999999, "Field Reading"=1.752265421591796e-05}, {0.0014734957045, "Field Reading"=7.086367144957606e-06}, {0.0014665331415, "Field Reading"=1.8102862099937696e-05}, {0.0014644652449999998, "Field Reading"=7.316505619558816e-06}, {0.001459879062, "Field Reading"=1.37617730508661e-05}, {0.001456597234, "Field Reading"=7.997778680662308e-06}, {0.001455313604, "Field Reading"=1.9441226029715573e-05}, {0.0014529164155, "Field Reading"=1.0715716208961658e-05}, {0.0014459223660000001, "Field Reading"=1.0707737364503455e-05}, {0.001443026579, "Field Reading"=9.286061057576923e-06}, {0.0014390227154999998, "Field Reading"=1.7041859386511388e-05}, {0.001435458936, "Field Reading"=1.0920769827263233e-05}, {0.0014284858615, "Field Reading"=1.3097238678707195e-05}, {0.0014155124364999998, "Field Reading"=1.4943301047674539e-05}, {0.0014111933845, "Field Reading"=5.8346849278326184e-06}, {0.0014089356844999997, "Field Reading"=1.6267991558672235e-05}, {0.001400876774, "Field Reading"=6.2157367659959844e-06}, {0.0013967058315, "Field Reading"=1.4893518977580172e-05}, {0.0013969721584999998, "Field Reading"=6.624033742801718e-06}, {0.0013922511495, "Field Reading"=1.2408363902223439e-05}, {0.0013878740965000001, "Field Reading"=1.1728994786990398e-05}, {0.0013784779875, "Field Reading"=1.6012598335679754e-05}, {0.001373894446, "Field Reading"=1.1607856045479023e-05}, {0.001376841956, "Field Reading"=1.3706169986026481e-05}, {0.0013736510590000002, "Field Reading"=1.2806127733243977e-05}, {0.0013650868689999997, "Field Reading"=8.195390358346867e-06}, {0.0013547451064999999, "Field Reading"=1.6565652587357594e-05}, {0.0013496873084999999, "Field Reading"=8.17962273174124e-06}, {0.001344070701, "Field Reading"=1.598311850023392e-05}, {0.0013365678835, "Field Reading"=1.68947157592058e-05}, {0.0013371844205000002, "Field Reading"=6.9113858577387e-06}, {0.0013289714789999998, "Field Reading"=1.6095504394402362e-05}, {0.0013241351944999996, "Field Reading"=8.708982244850283e-06}, {0.0013160219430000003, "Field Reading"=1.4995882937862019e-05}, {0.0013141926445, "Field Reading"=7.715603867966122e-06}, {0.001307578675, "Field Reading"=1.0508798844202823e-05}, {0.0013072095634999998, "Field Reading"=1.0844911550062126e-05}, {0.0013007955015, "Field Reading"=1.27924273437336e-05}, {0.0012968136035, "Field Reading"=1.2856378064505285e-05}, {0.0012935500455000001, "Field Reading"=4.230795106372986e-06}, {0.0012972608515, "Field Reading"=1.3137213193110304e-05}, {0.0012898972325000003, "Field Reading"=1.3386747104222238e-05}, {0.001282799791, "Field Reading"=7.931104461381083e-06}, {0.0012709697255000002, "Field Reading"=1.799425202500836e-05}, {0.0012674436765, "Field Reading"=9.058727595366937e-06}, {0.0012606737239999998, "Field Reading"=1.0991184753544291e-05}, {0.0012579929204999999, "Field Reading"=1.3934598114181036e-05}, {0.001257769553, "Field Reading"=7.958533117224735e-06}, {0.0012507587465, "Field Reading"=1.0091830908220513e-05}, {0.0012441302714999998, "Field Reading"=1.4247708625554687e-05}, {0.0012384482184999998, "Field Reading"=9.747850679960959e-06}, {0.0012301233445, "Field Reading"=1.0846592102338135e-05}, {0.0012257213105, "Field Reading"=1.2380409549105704e-05}, {0.0012199451029999996, "Field Reading"=1.2459487570359668e-05}, {0.00121674966, "Field Reading"=1.2684137656347864e-05}, {0.00121188588, "Field Reading"=8.670677469322843e-06}, {0.001206654942, "Field Reading"=1.2826265866859648e-05}, {0.001199749241, "Field Reading"=6.511686859953422e-06}, {0.0011963611185000001, "Field Reading"=1.621785476502402e-05}, {0.001191784512, "Field Reading"=3.876825454896724e-06}, {0.0011878949605, "Field Reading"=1.3553472395926025e-05}, {0.0011869933520000002, "Field Reading"=7.333818291110411e-06}, {0.00117880068, "Field Reading"=1.0887599025299673e-05}, {0.0011744038685, "Field Reading"=7.94010483980311e-06}, {0.0011652005910000002, "Field Reading"=1.4490920986637596e-05}, {0.0011613018139999998, "Field Reading"=9.394784663816004e-06}, {0.0011535013555, "Field Reading"=1.2352250452009829e-05}, {0.0011467069405000003, "Field Reading"=6.896661231107692e-06}, {0.0011455151755, "Field Reading"=7.337761001842288e-06}, {0.001138521796, "Field Reading"=1.0239089491114106e-05}, {0.0011344590175, "Field Reading"=1.0573325002691123e-05}, {0.0011261552115, "Field Reading"=8.647540631327389e-06}, {0.001123679251, "Field Reading"=1.3259501601164966e-05}, {0.0011187343909999999, "Field Reading"=6.326004309996491e-06}, {0.0011086951435000003, "Field Reading"=1.2644020368811997e-05}, {0.001106627641, "Field Reading"=4.558805388483696e-06}, {0.0010993935174999996, "Field Reading"=1.2280118637594773e-05}, {0.001095817554, "Field Reading"=6.209356935908581e-06}, {0.001092260756, "Field Reading"=1.1587590846080101e-05}, {0.0010857331680000002, "Field Reading"=8.053498732745852e-06}, {0.0010781649865000001, "Field Reading"=1.2595557021803393e-05}, {0.0010742738775, "Field Reading"=1.002251459845027e-05}, {0.0010700963025, "Field Reading"=1.1567215184584843e-05}, {0.0010665929600000002, "Field Reading"=9.71690253925762e-06}, {0.0010569922154999999, "Field Reading"=1.218375093526966e-05}, {0.001052063153, "Field Reading"=9.412420221769136e-06}, {0.001054387774, "Field Reading"=1.1036677157356432e-05}, {0.0010472023089999997, "Field Reading"=7.253528608289024e-06}, {0.0010405355485, "Field Reading"=8.654358204837474e-06}, {0.00103364433, "Field Reading"=1.4066022161534706e-05}, {0.0010263511880000001, "Field Reading"=5.95073368399531e-06}, {0.0010217420560000002, "Field Reading"=1.5003308761668754e-05}, {0.001019685314, "Field Reading"=7.241222740961668e-06}, {0.0010146316265, "Field Reading"=1.052694464691209e-05}, {0.0010164390084999998, "Field Reading"=8.865500178044464e-06}, {0.0010093353995, "Field Reading"=1.333555917138908e-05}, {0.0010006424937, "Field Reading"=1.16756554554672e-05}, {0.0009976462624000002, "Field Reading"=9.17628912574239e-06}, {0.0009889121786500004, "Field Reading"=7.667953510492475e-06}, {0.00098706200195, "Field Reading"=1.1473466670545638e-05}, {0.0009864765528500002, "Field Reading"=1.1952881928835212e-05}, {0.0009799007551999999, "Field Reading"=5.415796419232324e-06}, {0.0009807753594499998, "Field Reading"=1.2382709902382248e-05}, {0.0009742490892, "Field Reading"=1.0997355800995225e-05}, {0.0009681352198999998, "Field Reading"=1.0849337570594738e-05}, {0.0009649200989, "Field Reading"=1.2547072071289216e-05}, {0.0009592618809000002, "Field Reading"=8.546875891738046e-06}, {0.00094728407575, "Field Reading"=9.42409333615767e-06}, {0.0009437529853499998, "Field Reading"=1.241581201908061e-05}, {0.0009367892201999999, "Field Reading"=6.490097232182258e-06}, {0.00093690484695, "Field Reading"=9.305276824250138e-06}, {0.0009324354316999999, "Field Reading"=1.4455472085049554e-05}, {0.0009240299081999999, "Field Reading"=8.676186081900471e-06}, {0.0009163507952, "Field Reading"=1.0472650720532355e-05}, {0.000921669722, "Field Reading"=7.028853036116987e-06}, {0.00091520590965, "Field Reading"=1.1038784837914195e-05}, {0.0009158302097999999, "Field Reading"=1.2499381107046888e-05}, {0.0009042793933, "Field Reading"=7.999778970916443e-06}, {0.00090325085545, "Field Reading"=1.2707714731054025e-05}, {0.0008940475468000002, "Field Reading"=5.696700663056554e-06}, {0.0008881921163000001, "Field Reading"=1.3317352526367103e-05}, {0.0008792969681, "Field Reading"=1.1449125281013001e-05}, {0.0008766031075499999, "Field Reading"=8.067802902419195e-06}, {0.0008658052817500002, "Field Reading"=1.2494378459720566e-05}, {0.0008607013913000001, "Field Reading"=8.757506803237827e-06}, {0.0008550983522000001, "Field Reading"=7.979550494251882e-06}, {0.00084834499655, "Field Reading"=1.1637877057976928e-05}, {0.0008441038542999999, "Field Reading"=8.707482712389476e-06}, {0.0008384987585000001, "Field Reading"=1.1414437199685754e-05}, {0.00083580359865, "Field Reading"=9.92783908795231e-06}, {0.0008313148593, "Field Reading"=9.987285704363987e-06}, {0.0008253860362499999, "Field Reading"=1.220082390947404e-05}, {0.0008201507233500001, "Field Reading"=9.775538861908423e-06}, {0.00080883225105, "Field Reading"=6.848506313785722e-06}, {0.00080730096785, "Field Reading"=9.658705857926318e-06}, {0.00079779620115, "Field Reading"=1.1161719714964172e-05}, {0.0007978070924499999, "Field Reading"=7.576893315859874e-06}, {0.0007912592465999999, "Field Reading"=9.135224842990904e-06}, {0.0007837346065500001, "Field Reading"=1.1429223899565665e-05}, {0.00077881317535, "Field Reading"=9.356914527443012e-06}, {0.0007730561324499999, "Field Reading"=8.044243410483363e-06}, {0.0007659974883, "Field Reading"=1.1968541586438558e-05}, {0.0007599484890500002, "Field Reading"=5.766670320976711e-06}, {0.0007554092201500001, "Field Reading"=1.0290206226262234e-05}, {0.0007568849260499999, "Field Reading"=9.095609970425388e-06}, {0.00074690365015, "Field Reading"=7.428351278092278e-06}, {0.0007412911153999999, "Field Reading"=1.2211144747880274e-05}, {0.0007388490718999999, "Field Reading"=7.119754195100964e-06}, {0.00073184585735, "Field Reading"=1.11973674743817e-05}, {0.0007289355012, "Field Reading"=9.87201156601368e-06}, {0.0007260416204499999, "Field Reading"=9.893571725350646e-06}, {0.0007160901174, "Field Reading"=1.0966974229535269e-05}, {0.00070773075435, "Field Reading"=8.36483154859936e-06}, {0.00070562201435, "Field Reading"=1.1135745609001538e-05}, {0.0007005231824, "Field Reading"=7.792111761910039e-06}, {0.0006984861534500001, "Field Reading"=1.112326620533237e-05}, {0.0006913369775500001, "Field Reading"=8.906384794122927e-06}, {0.00068368938035, "Field Reading"=7.692500139277996e-06}, {0.0006827128907, "Field Reading"=1.1168780160980318e-05}, {0.0006785491257000001, "Field Reading"=9.884474762989764e-06}, {0.0006703142008, "Field Reading"=7.476499449316608e-06}, {0.00066343855645, "Field Reading"=1.0671681694929994e-05}, {0.0006575070245499998, "Field Reading"=7.4347658191749286e-06}, {0.0006511912740000001, "Field Reading"=9.425657051979277e-06}, {0.0006441312950999999, "Field Reading"=7.335231935722649e-06}, {0.0006414379744, "Field Reading"=1.1662581651496823e-05}, {0.00063651898405, "Field Reading"=6.333514465013529e-06}, {0.0006290483447500001, "Field Reading"=1.0445958662672352e-05}, {0.00062158186175, "Field Reading"=7.261656284234062e-06}, {0.00061594993845, "Field Reading"=7.989757889991673e-06}, {0.00061236428065, "Field Reading"=8.961528298010006e-06}, {0.00060375337885, "Field Reading"=7.694962223570544e-06}, {0.00059621971245, "Field Reading"=1.1940420080469981e-05}, {0.0005919004317, "Field Reading"=7.0548124548985455e-06}, {0.0005857217634000001, "Field Reading"=8.765203101488766e-06}, {0.0005791150372000001, "Field Reading"=8.250255887268706e-06}, {0.0005752629281999999, "Field Reading"=9.242197266516861e-06}, {0.0005699006454000001, "Field Reading"=9.316912086921557e-06}, {0.0005616036655000001, "Field Reading"=9.983684789127442e-06}, {0.0005558463523, "Field Reading"=7.379838030630408e-06}, {0.0005448341282499999, "Field Reading"=9.133549323107993e-06}, {0.0005419575418000001, "Field Reading"=7.243809280707957e-06}, {0.0005382379248499999, "Field Reading"=1.131671442135203e-05}, {0.0005344668938, "Field Reading"=6.581627717251058e-06}, {0.0005244464583000001, "Field Reading"=1.004401822667721e-05}, {0.0005216683419, "Field Reading"=6.2669344348143284e-06}, {0.0005172088394500001, "Field Reading"=8.88869297030887e-06}, {0.0005098693518499999, "Field Reading"=7.014837917272097e-06}, {0.00049886621595, "Field Reading"=1.011836746000351e-05}, {0.0004960390570499999, "Field Reading"=7.467175666597576e-06}, {0.0004922772224000001, "Field Reading"=9.065659621261306e-06}, {0.00048465027175000004, "Field Reading"=7.82137970283589e-06}, {0.00047901529220000004, "Field Reading"=9.687548703450598e-06}, {0.000474211401, "Field Reading"=7.570586234472122e-06}, {0.00046536972845, "Field Reading"=1.098327646496162e-05}, {0.0004611677763999999, "Field Reading"=7.2229414652975575e-06}, {0.00045522123724999993, "Field Reading"=9.251151423262948e-06}, {0.00045021791485, "Field Reading"=7.265622449362038e-06}, {0.00044626679465, "Field Reading"=1.0214845778945212e-05}, {0.00044156144705000003, "Field Reading"=7.279197954522579e-06}, {0.0004357334483000001, "Field Reading"=8.74300238542749e-06}, {0.00042780705335000003, "Field Reading"=8.708777475030662e-06}, {0.00041766146795, "Field Reading"=9.268214168304002e-06}, {0.0004113853006499999, "Field Reading"=8.279864389911588e-06}, {0.00040281951819999995, "Field Reading"=9.349697911305399e-06}, {0.00039788142904999995, "Field Reading"=8.553568677090712e-06}, {0.00039139665024999997, "Field Reading"=8.35701873438238e-06}, {0.00038832555510000006, "Field Reading"=8.508901794612005e-06}, {0.00038026128380000006, "Field Reading"=8.924006533360109e-06}, {0.0003764893644, "Field Reading"=9.159161335270996e-06}, {0.00037596292550000007, "Field Reading"=7.948058516495947e-06}, {0.00036894467525, "Field Reading"=9.031833740625616e-06}, {0.0003597119468, "Field Reading"=8.447065074021638e-06}, {0.00035069281800000003, "Field Reading"=9.847468588013626e-06}, {0.00034670346585, "Field Reading"=7.046734671994317e-06}, {0.00034549796655000003, "Field Reading"=1.0163653804944002e-05}, {0.0003450545487, "Field Reading"=7.480561026258937e-06}, {0.00033551175375, "Field Reading"=9.073095802267394e-06}, {0.00032746944515, "Field Reading"=7.767711826671478e-06}, {0.00032069032435000003, "Field Reading"=9.051940298970106e-06}, {0.00031907733195, "Field Reading"=8.09792989830245e-06}, {0.00031349352920000004, "Field Reading"=9.032615603870342e-06}, {0.0003068844543, "Field Reading"=9.195456597325915e-06}, {0.0002976679609, "Field Reading"=9.083569010978934e-06}, {0.00028997314390000005, "Field Reading"=9.105037977474842e-06}, {0.0002822417988499999, "Field Reading"=1.0817725242627848e-05}, {0.00027856539714999994, "Field Reading"=8.294038871944025e-06}, {0.0002756308612, "Field Reading"=9.488759591378838e-06}, {0.00027053675769999995, "Field Reading"=8.42286336033488e-06}, {0.00026473204595000004, "Field Reading"=1.0616612488305245e-05}, {0.00025843440024999996, "Field Reading"=8.52039526536792e-06}, {0.00025232634085, "Field Reading"=9.040092319227756e-06}, {0.00024696605939999994, "Field Reading"=1.0130795585889413e-05}, {0.00023728632205, "Field Reading"=9.69308163379321e-06}, {0.00023007721425, "Field Reading"=9.372252617142177e-06}, {0.00022658243825, "Field Reading"=1.0063987026550166e-05}, {0.00022278867680000002, "Field Reading"=9.573266136591687e-06}, {0.00021816389565, "Field Reading"=1.0367696494256549e-05}, {0.00021204833639999998, "Field Reading"=9.5636017844066e-06}, {0.00021146626760000002, "Field Reading"=1.1731461487718655e-05}, {0.0002108107251, "Field Reading"=9.752006576393727e-06}, {0.00020708452405000002, "Field Reading"=1.1847826012272043e-05}, {0.00019848133049999998, "Field Reading"=9.774628043136221e-06}, {0.00019234139270000002, "Field Reading"=1.1090973726713319e-05}, {0.00018527486454999998, "Field Reading"=1.0578934347660143e-05}, {0.00018058074714999997, "Field Reading"=1.145170312108404e-05}, {0.0001764918464, "Field Reading"=1.2733255476727721e-05}, {0.00017345773179999998, "Field Reading"=1.0965919136503228e-05}, {0.00017412942404999997, "Field Reading"=1.2833532792420877e-05}, {0.00016752787079999998, "Field Reading"=1.1537755964684765e-05}, {0.00016390472585, "Field Reading"=1.4058604632967103e-05}, {0.00015893333165000002, "Field Reading"=1.3525749310590882e-05}, {0.00015733645934999999, "Field Reading"=1.2750969115761529e-05}, {0.00015445027835, "Field Reading"=1.493992901560813e-05}, {0.00015224330005000002, "Field Reading"=1.2534901890684785e-05}, {0.00015107007170000002, "Field Reading"=1.4654869395297748e-05}, {0.00014296859130000003, "Field Reading"=1.4491515559368466e-05}, {0.00014101790225000004, "Field Reading"=1.4612258968164335e-05}, {0.00013789251349999998, "Field Reading"=1.4985214074225936e-05}, {0.0001333535397, "Field Reading"=1.2910825406256663e-05}, {0.00013293488295, "Field Reading"=1.5204263118022852e-05}, {0.00012824479430000003, "Field Reading"=1.5814987757713907e-05}, {0.00012001902010000001, "Field Reading"=1.1946409871421038e-05}, {0.00011640474784999999, "Field Reading"=1.374178568139533e-05}, {0.00011164799804999998, "Field Reading"=1.2686777475368162e-05}, {0.0001114707303, "Field Reading"=1.2531683397771152e-05}, {0.00010370220725, "Field Reading"=1.2373558795592057e-05}, {9.6105127615e-05, "Field Reading"=1.1405443098621103e-05}, {9.3427342245e-05, "Field Reading"=9.114920667213266e-06}, {8.631985702e-05, "Field Reading"=8.55715381226974e-06}, {8.2231697615e-05, "Field Reading"=7.919632084505655e-06}, {7.373111064e-05, "Field Reading"=6.0220271023881185e-06}, {6.615270785000001e-05, "Field Reading"=4.576748734898483e-06}, {4.7618336285e-05, "Field Reading"=2.4760765618784777e-06}, {8.088163554999999e-06, "Field Reading"=8.522804838208432e-07}, {-0.00031203726999999993, "Field Reading"=9.340031444244631e-08}, {-0.0004431156068, "Field Reading"=1.5599650025926086e-06}, {-0.00047447420259999994, "Field Reading"=3.3699081066143133e-06}, {-0.0004891067322000001, "Field Reading"=5.251639511591731e-06}, {-0.0004965016292500001, "Field Reading"=6.753188658649841e-06}, {-0.0005065220433, "Field Reading"=8.05029568075816e-06}, {-0.0005119405476000001, "Field Reading"=8.996646103928022e-06}, {-0.0005181177034000002, "Field Reading"=9.586125099466969e-06}, {-0.0005233375587, "Field Reading"=1.0780593271476432e-05}, {-0.0005264042754499999, "Field Reading"=1.151068450862685e-05}, {-0.00053110047595, "Field Reading"=1.2726641422828874e-05}, {-0.00053324047765, "Field Reading"=1.4096974813626132e-05}, {-0.00053687322925, "Field Reading"=1.168803560424343e-05}, {-0.0005389412610000001, "Field Reading"=1.5380911429792524e-05}, {-0.0005462915548999999, "Field Reading"=1.3641306492412249e-05}, {-0.0005491646896500001, "Field Reading"=1.7598769051749004e-05}, {-0.0005526108069500001, "Field Reading"=1.2871009431175905e-05}, {-0.0005570165338000001, "Field Reading"=1.387574726991729e-05}, {-0.0005586084761499998, "Field Reading"=1.3712948314379189e-05}, {-0.00056355646615, "Field Reading"=1.4632613185113879e-05}, {-0.0005702242301500001, "Field Reading"=1.2208181277474454e-05}, {-0.00057438249675, "Field Reading"=1.3993001530491093e-05}, {-0.0005772129525, "Field Reading"=1.2319386830884628e-05}, {-0.0005802113718, "Field Reading"=1.3382369477296797e-05}, {-0.0005816963447500001, "Field Reading"=1.3705876328930594e-05}, {-0.00058789514975, "Field Reading"=1.3678003266414856e-05}, {-0.0005941986325, "Field Reading"=1.2839960748553288e-05}, {-0.000597252894, "Field Reading"=1.1076678146303071e-05}, {-0.0005966246987, "Field Reading"=1.1670866522169375e-05}, {-0.0005959692223999999, "Field Reading"=1.1329039807107005e-05}, {-0.0006060982143000001, "Field Reading"=1.1410436788769928e-05}, {-0.0006145074601, "Field Reading"=1.1049964827299401e-05}, {-0.0006193374012500001, "Field Reading"=1.1479732901485121e-05}, {-0.0006210421742499999, "Field Reading"=1.1355176813229608e-05}, {-0.000626744072, "Field Reading"=1.0176579758441679e-05}, {-0.0006321316623, "Field Reading"=9.184275869844095e-06}, {-0.0006380585723000001, "Field Reading"=1.0459377622380703e-05}, {-0.0006426511809000001, "Field Reading"=9.707573147759142e-06}, {-0.00064842313815, "Field Reading"=9.312624781346977e-06}, {-0.0006566046421499999, "Field Reading"=9.597042854592816e-06}, {-0.0006617673212500001, "Field Reading"=1.0542187621680919e-05}, {-0.0006677974469499999, "Field Reading"=9.777298158787781e-06}, {-0.00067432441115, "Field Reading"=9.216599093618808e-06}, {-0.0006748317891499999, "Field Reading"=9.045248712344223e-06}, {-0.00067757612315, "Field Reading"=8.181782834043983e-06}, {-0.00068409381025, "Field Reading"=1.0053248936070572e-05}, {-0.0006902701867499999, "Field Reading"=9.014760801380515e-06}, {-0.0006929725644999999, "Field Reading"=1.0522147956013759e-05}, {-0.0007008359415999999, "Field Reading"=8.39794631525331e-06}, {-0.00070618279725, "Field Reading"=1.020476411893954e-05}, {-0.0007109699488, "Field Reading"=8.157086041794205e-06}, {-0.0007161346874000001, "Field Reading"=9.809157487830533e-06}, {-0.00071664314305, "Field Reading"=7.72876700626727e-06}, {-0.0007222599683, "Field Reading"=7.753771393024295e-06}, {-0.0007286956131999999, "Field Reading"=1.0366002056919536e-05}, {-0.0007365894205000001, "Field Reading"=8.094947334995277e-06}, {-0.0007425676660500001, "Field Reading"=1.026857504729432e-05}, {-0.0007499141079000001, "Field Reading"=6.817369622943153e-06}, {-0.0007575060436999999, "Field Reading"=9.64939244699465e-06}, {-0.0007608931877, "Field Reading"=9.604007671349509e-06}, {-0.00076930784845, "Field Reading"=6.9181619479098136e-06}, {-0.0007781628024500001, "Field Reading"=9.116472059182675e-06}, {-0.00078172888895, "Field Reading"=1.0568158361127749e-05}, {-0.00078337772275, "Field Reading"=8.081886907257952e-06}, {-0.0007925322146000001, "Field Reading"=8.562368085556535e-06}, {-0.0007994605006000001, "Field Reading"=9.437470264147786e-06}, {-0.0008054270838500001, "Field Reading"=7.079640068413085e-06}, {-0.00081384801795, "Field Reading"=1.0902253918362219e-05}, {-0.00081610829425, "Field Reading"=7.2507309221227275e-06}, {-0.00082288074665, "Field Reading"=8.449941478288062e-06}, {-0.0008295853276, "Field Reading"=8.702255137506673e-06}, {-0.0008406569691, "Field Reading"=9.535617817911213e-06}, {-0.0008484793012500001, "Field Reading"=8.52094520817387e-06}, {-0.00085187527465, "Field Reading"=8.918533022298948e-06}, {-0.0008584232488500002, "Field Reading"=7.831317128053835e-06}, {-0.0008643170760499998, "Field Reading"=8.637448486295988e-06}, {-0.0008685804436, "Field Reading"=8.271575864909405e-06}, {-0.0008757553470499999, "Field Reading"=9.235830965976584e-06}, {-0.0008777516488, "Field Reading"=8.034566362783523e-06}, {-0.00088532026625, "Field Reading"=6.358317126980454e-06}, {-0.0008904377534499998, "Field Reading"=7.691825333984003e-06}, {-0.0008959099107999999, "Field Reading"=8.96988312322161e-06}, {-0.00090052076335, "Field Reading"=8.401521222725386e-06}, {-0.00090882224315, "Field Reading"=8.846826499402912e-06}, {-0.0009153773639999998, "Field Reading"=8.535674603093436e-06}, {-0.0009216683318000001, "Field Reading"=7.911130674820287e-06}, {-0.0009293472133, "Field Reading"=9.42216335567201e-06}, {-0.0009334509418999999, "Field Reading"=7.46810582605106e-06}, {-0.0009376995239000002, "Field Reading"=9.612634461992838e-06}, {-0.0009429223466000001, "Field Reading"=7.982128993384355e-06}, {-0.0009481757170000001, "Field Reading"=9.606787602183041e-06}, {-0.0009521188455500001, "Field Reading"=6.839542702034589e-06}, {-0.0009625084431, "Field Reading"=1.0053375161154321e-05}, {-0.0009687315084000002, "Field Reading"=1.0000198882713586e-05}, {-0.0009724786526499999, "Field Reading"=8.230584226840804e-06}, {-0.00098003340505, "Field Reading"=8.530208769113411e-06}, {-0.0009853039495500001, "Field Reading"=8.77944225374735e-06}, {-0.0009908962838999999, "Field Reading"=8.02944926499699e-06}, {-0.0009986952382, "Field Reading"=9.317842156444721e-06}, {-0.0010041144209999998, "Field Reading"=7.22863595579311e-06}, {-0.001002674158, "Field Reading"=1.0350798604682632e-05}, {-0.0010133611645, "Field Reading"=7.302538953944351e-06}, {-0.001016922732, "Field Reading"=1.040540565609174e-05}, {-0.0010242121479999999, "Field Reading"=6.786233430326999e-06}, {-0.0010286114905, "Field Reading"=9.378011559618059e-06}, {-0.0010333265045, "Field Reading"=7.471698682552988e-06}, {-0.0010404976735, "Field Reading"=8.132945424821094e-06}, {-0.0010431231284999999, "Field Reading"=8.077137423576924e-06}, {-0.0010526726995, "Field Reading"=9.000828580325923e-06}, {-0.0010608102004999998, "Field Reading"=7.79951702819659e-06}, {-0.001066157949, "Field Reading"=8.026787828282276e-06}, {-0.0010660587799999999, "Field Reading"=9.292933839621613e-06}, {-0.001071659163, "Field Reading"=6.51723890933294e-06}, {-0.0010740595745, "Field Reading"=9.88075030403542e-06}, {-0.001081231224, "Field Reading"=8.165419998292393e-06}, {-0.0010889585195, "Field Reading"=9.540229442005787e-06}, {-0.0010936563135000002, "Field Reading"=8.665690390146306e-06}, {-0.0011004628195000002, "Field Reading"=9.14266992905204e-06}, {-0.001104228082, "Field Reading"=9.068034603601546e-06}, {-0.0011111721555000001, "Field Reading"=9.258650076136835e-06}, {-0.0011157116515, "Field Reading"=8.794150582877372e-06}, {-0.001117935175, "Field Reading"=1.0049928602301134e-05}, {-0.0011229755575, "Field Reading"=9.26964267985305e-06}, {-0.001125548458, "Field Reading"=9.512963423684153e-06}, {-0.0011358785320000001, "Field Reading"=1.162298707303496e-05}, {-0.0011401705135, "Field Reading"=8.673920562266882e-06}, {-0.0011436530790000002, "Field Reading"=1.026363880447038e-05}, {-0.0011528469005, "Field Reading"=7.343341732879041e-06}, {-0.001158585503, "Field Reading"=1.1221438357709664e-05}, {-0.001163272579, "Field Reading"=6.788543901191646e-06}, {-0.0011652281590000002, "Field Reading"=1.1163538168206555e-05}, {-0.0011696641304999999, "Field Reading"=6.987608150535051e-06}, {-0.0011769647225000001, "Field Reading"=1.1397508506035563e-05}, {-0.0011826203915, "Field Reading"=6.6791406969640645e-06}, {-0.0011856012369999998, "Field Reading"=1.1791918650940167e-05}, {-0.0011923716495, "Field Reading"=6.10201255176998e-06}, {-0.0011950962400000002, "Field Reading"=1.127183683879996e-05}, {-0.0011993509359999998, "Field Reading"=7.3168465124108586e-06}, {-0.0012063977555000001, "Field Reading"=1.0673139458316081e-05}, {-0.001211625169, "Field Reading"=8.42668371261418e-06}, {-0.0012185852359999998, "Field Reading"=8.924242304208964e-06}, {-0.0012296836459999999, "Field Reading"=9.214907534843816e-06}, {-0.0012341990425, "Field Reading"=1.029757573456139e-05}, {-0.0012360992634999999, "Field Reading"=1.028327582601235e-05}, {-0.0012451840445000003, "Field Reading"=9.721115565811265e-06}, {-0.0012518802965000003, "Field Reading"=1.0870160833599113e-05}, {-0.001254286168, "Field Reading"=8.10702674211348e-06}, {-0.0012614180595, "Field Reading"=1.0709583241200152e-05}, {-0.0012700799079999998, "Field Reading"=8.080288214879785e-06}, {-0.0012728665429999999, "Field Reading"=1.1543837929010972e-05}, {-0.0012752597895, "Field Reading"=7.649280247935341e-06}, {-0.001280031124, "Field Reading"=1.3989167347468871e-05}, {-0.0012910045725, "Field Reading"=7.4411341155019085e-06}, {-0.0012938469575000003, "Field Reading"=1.222721223100134e-05}, {-0.0012988768950000004, "Field Reading"=7.068543596233621e-06}, {-0.0013053452874999998, "Field Reading"=1.201341201714014e-05}, {-0.0013088561730000001, "Field Reading"=5.600173823206697e-06}, {-0.0013117916075, "Field Reading"=1.0006690101617936e-05}, {-0.0013136245115, "Field Reading"=7.92740379550217e-06}, {-0.0013194145515000003, "Field Reading"=1.1307931637499589e-05}, {-0.0013252378065, "Field Reading"=1.0489955813420106e-05}, {-0.0013309848304999998, "Field Reading"=1.0354713769623458e-05}, {-0.0013344076250000002, "Field Reading"=9.676833762668265e-06}, {-0.0013403081224999999, "Field Reading"=1.0706859479632934e-05}, {-0.001344153754, "Field Reading"=9.53613815985326e-06}, {-0.001353717271, "Field Reading"=1.2153004599260104e-05}, {-0.0013589400385, "Field Reading"=1.1147930313234938e-05}, {-0.0013651392094999998, "Field Reading"=1.0233736083788055e-05}, {-0.0013703597609999998, "Field Reading"=1.2101840809088374e-05}, {-0.0013746799340000001, "Field Reading"=1.0434330130862396e-05}, {-0.0013767243149999998, "Field Reading"=8.965578917510663e-06}, {-0.0013811278984999999, "Field Reading"=1.2383490382104567e-05}, {-0.0013862338874999999, "Field Reading"=1.150927969297647e-05}, {-0.001390332012, "Field Reading"=8.883236654722128e-06}, {-0.0013968710690000002, "Field Reading"=1.0564235269575693e-05}, {-0.0014023384790000002, "Field Reading"=1.1545589087214473e-05}, {-0.001404902543, "Field Reading"=9.413346111306029e-06}, {-0.0014156881870000001, "Field Reading"=9.955146596702317e-06}, {-0.0014200097435, "Field Reading"=8.982312529982237e-06}, {-0.0014251782900000002, "Field Reading"=9.139181004488435e-06}, {-0.0014309121145, "Field Reading"=8.758345662525561e-06}, {-0.001437344702, "Field Reading"=9.536769128246045e-06}, {-0.0014424840345, "Field Reading"=1.2408218410110771e-05}, {-0.001445603983, "Field Reading"=7.121531323396436e-06}, {-0.001447866259, "Field Reading"=1.1823908162158577e-05}, {-0.0014513563639999998, "Field Reading"=1.2069148463537112e-05}, {-0.0014609864175000001, "Field Reading"=1.0789381957184024e-05}, {-0.0014633654675, "Field Reading"=1.3637925928838184e-05}, {-0.001470391416, "Field Reading"=8.467902917866855e-06}, {-0.00147624995, "Field Reading"=8.713320040370468e-06}, {-0.001478446956, "Field Reading"=1.0141676924633733e-05}, {-0.001484861428, "Field Reading"=1.056909975094943e-05}, {-0.0014958812725000001, "Field Reading"=7.936935666852078e-06}, {-0.0014965657290000002, "Field Reading"=1.0495855235198695e-05}, {-0.001502919273, "Field Reading"=8.910048050023552e-06}, {-0.0015083071505, "Field Reading"=7.914652202479758e-06}, {-0.0015100368374999999, "Field Reading"=6.259399103273022e-06}, {-0.0015175668834999999, "Field Reading"=7.334045182579369e-06}, {-0.0015203300695000002, "Field Reading"=8.864672725701856e-06}, {-0.0015301117994999999, "Field Reading"=8.150423791799691e-06}, {-0.0015376529015, "Field Reading"=6.678676832102852e-06}, {-0.0015407987600000003, "Field Reading"=9.696111671223899e-06}, {-0.0015464850944999998, "Field Reading"=1.1858675346692954e-05}, {-0.0015503071805, "Field Reading"=1.1249500764863822e-05}, {-0.001556784684, "Field Reading"=8.7270056262674e-06}, {-0.001561760317, "Field Reading"=1.132128500969807e-05}, {-0.0015630432335, "Field Reading"=1.2179842735862834e-05}, {-0.001568771859, "Field Reading"=1.3204072479362346e-05}, {-0.0015781199194999998, "Field Reading"=6.905292575758025e-06}, {-0.0015834545165, "Field Reading"=1.2114250524009491e-05}, {-0.0015888747935000002, "Field Reading"=1.0990137997176201e-05}, {-0.0015943893824999999, "Field Reading"=1.2244038741460848e-05}, {-0.0015986649615000001, "Field Reading"=9.867055344455419e-06}, {-0.0016009483040000001, "Field Reading"=1.388783918041585e-05}, {-0.0016047094665, "Field Reading"=7.924281983853592e-06}, {-0.0016109609995, "Field Reading"=9.525383017697709e-06}, {-0.0016163201465000001, "Field Reading"=6.295675525473667e-06}, {-0.0016193981280000001, "Field Reading"=1.2418835825222594e-05}, {-0.0016235575870000001, "Field Reading"=7.241022443188336e-06}, {-0.001631376714, "Field Reading"=1.1414443865009429e-05}, {-0.0016416887995000001, "Field Reading"=1.3856989126669188e-05}, {-0.0016460461620000002, "Field Reading"=1.2883594888902582e-05}, {-0.0016493999085000002, "Field Reading"=1.3451361579915418e-05}, {-0.0016543726325000002, "Field Reading"=1.0197524054106919e-05}, {-0.0016580187500000003, "Field Reading"=8.35915914435297e-06}, {-0.0016608696945000002, "Field Reading"=1.2038124513587692e-05}, {-0.0016644504264999999, "Field Reading"=1.2073756152549215e-05}, {-0.0016743514875000001, "Field Reading"=1.4163431524276783e-05}, {-0.001680846064, "Field Reading"=1.1721643692782217e-05}, {-0.001680180823, "Field Reading"=1.4522736663586213e-05}, {-0.0016891537449999997, "Field Reading"=1.000893210270047e-05}, {-0.0016959669994999998, "Field Reading"=1.1950982549190453e-05}, {-0.0017038495714999998, "Field Reading"=9.666369362675669e-06}, {-0.0017068791164999999, "Field Reading"=1.0290538132586155e-05}, {-0.001712292553, "Field Reading"=1.55531491764059e-05}, {-0.0017191365170000001, "Field Reading"=6.163208684575526e-06}, {-0.0017203984770000004, "Field Reading"=1.3588408558436078e-05}, {-0.0017253935954999998, "Field Reading"=6.4677406574536974e-06}, {-0.0017318057010000001, "Field Reading"=8.447796579612885e-06}, {-0.0017341460054999998, "Field Reading"=8.04828399573741e-06}, {-0.0017385906875, "Field Reading"=7.953355703600843e-06}, {-0.0017443079605000001, "Field Reading"=5.743648506866208e-06}, {-0.0017471709909999997, "Field Reading"=5.48590727511866e-06}, {-0.001750861947, "Field Reading"=8.023366701230126e-06}, {-0.0017534107624999997, "Field Reading"=1.4833661288978803e-05}, {-0.0017603070280000001, "Field Reading"=9.603059725986412e-06}, {-0.001764742602, "Field Reading"=1.7929399276795733e-05}, {-0.0017691532744999999, "Field Reading"=6.3563871288555276e-06}, {-0.0017741060039999999, "Field Reading"=1.501973943116676e-05}, {-0.001777655756, "Field Reading"=6.869160584141547e-06}, {-0.0017825162375000002, "Field Reading"=1.2056375635818308e-05}, {-0.0017885220945000001, "Field Reading"=1.642451658977561e-05}, {-0.0017914973770000002, "Field Reading"=6.719746034808603e-06}, {-0.0017977745674999997, "Field Reading"=1.7805760018497386e-05}, {-0.001801836109, "Field Reading"=8.97764211057813e-06}, {-0.0018092166519999998, "Field Reading"=1.5135881807316772e-05}, {-0.0018143644185000002, "Field Reading"=8.704393062544215e-06}, {-0.0018189728425, "Field Reading"=1.2416876104869778e-05}, {-0.0018223028215000002, "Field Reading"=1.0307651626472604e-05}, {-0.0018264975419999998, "Field Reading"=1.3588915931050962e-05}, {-0.0018297345360000002, "Field Reading"=7.542684981570812e-06}, {-0.0018376653684999997, "Field Reading"=1.466443025875735e-05}, {-0.0018409885535, "Field Reading"=8.667490662707144e-06}, {-0.0018439941659999996, "Field Reading"=1.8977797265170493e-05}, {-0.0018537341870000002, "Field Reading"=7.960870183466045e-06}, {-0.001859281325, "Field Reading"=1.7596121309015976e-05}, {-0.0018625259804999998, "Field Reading"=4.664985640037273e-06}, {-0.0018678461475, "Field Reading"=1.769330303102707e-05}, {-0.001871559871, "Field Reading"=4.364809569647222e-06}, {-0.0018766502185000003, "Field Reading"=1.5867801299378025e-05}, {-0.0018819159935, "Field Reading"=1.398324744367411e-05}, {-0.0018853722179999997, "Field Reading"=6.609614539686083e-06}, {-0.001888117514, "Field Reading"=1.1049834308553432e-05}, {-0.0018970659275000003, "Field Reading"=1.2006070876482268e-05}, {-0.0019015492525000003, "Field Reading"=1.1311678876601407e-05}, {-0.0019069758595, "Field Reading"=1.1735161252899554e-05}, {-0.0019104908274999999, "Field Reading"=1.3773417917656903e-05}, {-0.0019134597475000004, "Field Reading"=9.817988058013217e-06}, {-0.0019170247744999998, "Field Reading"=5.5475406517366205e-06}, {-0.0019216890985000001, "Field Reading"=1.6518864383668388e-05}, {-0.001925480497, "Field Reading"=8.07650608714714e-06}, {-0.0019310675759999997, "Field Reading"=1.81041161084976e-05}, {-0.0019390837075, "Field Reading"=9.568908174406485e-06}, {-0.0019433324869999997, "Field Reading"=1.813623370449535e-05}, {-0.0019506690995000002, "Field Reading"=8.780171145913223e-06}, {-0.001958867488, "Field Reading"=1.6029862249452948e-05}, {-0.0019637680994999997, "Field Reading"=1.2253495405595064e-05}, {-0.0019661004000000007, "Field Reading"=7.5557372216271175e-06}, {-0.001972397318, "Field Reading"=1.9373578095147194e-05}, {-0.0019756450445, "Field Reading"=1.4064569403677659e-05}, {-0.0019792207135000003, "Field Reading"=9.284463736707293e-06}, {-0.0019847661455, "Field Reading"=1.4202159786271747e-05}, {-0.0019895345655, "Field Reading"=1.1107140492957775e-05}, {-0.00199533579, "Field Reading"=1.9367144370174343e-05}, {-0.0019978300919999996, "Field Reading"=1.0027918784716801e-05}, {-0.0020014526555, "Field Reading"=1.4795147302132685e-05}, {-0.0020093011694999998, "Field Reading"=1.166451327147869e-05}, {-0.0020132605230000003, "Field Reading"=1.3243296188513057e-05}, {-0.0020184218760000002, "Field Reading"=1.4075797219037401e-05}, {-0.0020218959709999997, "Field Reading"=1.2867523151846156e-05}, {-0.0020257192415, "Field Reading"=1.4283358143549602e-05}, {-0.002031346276, "Field Reading"=6.372088523117207e-06}, {-0.0020322277155, "Field Reading"=1.6091549408094542e-05}, {-0.0020364816525000004, "Field Reading"=8.086227199257814e-06}, {-0.002042609889, "Field Reading"=1.8027178741110802e-05}, {-0.002045313605, "Field Reading"=6.234105608687719e-06}, {-0.0020486091915, "Field Reading"=1.2688964729805642e-05}, {-0.0020527189510000004, "Field Reading"=5.248626243149417e-06}, {-0.0020576646070000005, "Field Reading"=1.7520501899380802e-05}, {-0.0020646581015000003, "Field Reading"=5.036074934391022e-06}, {-0.0020683215144999996, "Field Reading"=1.595281076792403e-05}, {-0.0020703297770000005, "Field Reading"=7.649488847989299e-06}, {-0.002072542353, "Field Reading"=1.6952454165185355e-05}, {-0.00207905954, "Field Reading"=8.526727115979576e-06}, {-0.002079054116, "Field Reading"=2.0803525197653414e-05}, {-0.002084624442, "Field Reading"=8.210125507079418e-06}, {-0.0020935904525, "Field Reading"=1.2074480976024989e-05}, {-0.0020979551465, "Field Reading"=1.0494567013701489e-05}, {-0.0021015473665, "Field Reading"=1.2941680194973117e-05}, {-0.002104104307, "Field Reading"=1.6098280625825472e-05}, {-0.002107640578, "Field Reading"=1.0574004274378893e-05}, {-0.0021140479824999997, "Field Reading"=1.3908412165814616e-05}, {-0.002119767525, "Field Reading"=1.460409450668384e-05}, {-0.0021221912375, "Field Reading"=1.402153586924527e-05}, {-0.002127163972, "Field Reading"=7.125231924569935e-06}, {-0.0021325035915, "Field Reading"=1.639509777121526e-05}, {-0.0021391739079999997, "Field Reading"=7.358370302935656e-06}, {-0.0021455499954999998, "Field Reading"=1.7770808080950035e-05}, {-0.0021497235765, "Field Reading"=6.941112564522383e-06}, {-0.0021552409425, "Field Reading"=2.0184167438232853e-05}, {-0.002160739336, "Field Reading"=4.994465512890516e-06}, {-0.002166699126, "Field Reading"=2.3173056337643402e-05}, {-0.00217069716, "Field Reading"=5.042376211549365e-06}, {-0.0021781266294999997, "Field Reading"=1.789107471782907e-05}, {-0.0021796036155000004, "Field Reading"=1.7047416335970956e-05}, {-0.0021848448555, "Field Reading"=7.322148533670827e-06}, {-0.0021857902645, "Field Reading"=2.4426615391620698e-05}, {-0.0021872726050000003, "Field Reading"=1.1754263355219391e-05}, {-0.002196666813, "Field Reading"=1.7672056800517004e-05}, {-0.0022013766920000004, "Field Reading"=6.914010210132466e-06}]
  out "DC Voltage (V) 2":dbl=-0.0022013766920000004
  out "dI/dV (ohm) 2":dbl=6.914010210132466e-06
  out "dV (V) 2":dbl=5.034309826469514e-06
  out "dI (A) 2":dbl=3.480726954118042e-11
  in  "DC Voltage averaging 2":dbl=20.0 format="%#_13g"
  out "Vset (V) 2":dbl=-1.6999999999999718
  in  "MFLI Averaging (Device2)":dbl=20.0 format="%#_13g"
  out "File path 2":path=path "D:/Pranava/Data/STS/MA2479/004_MA2479_[Dev90]_40uV_33pA_7.919Hz_4thorder_300ms_0T_measureX_float_20xaverage.dat"
  in  "DC Current Limit (A)":dbl=0.0001 format="%#_13g"
  in  "Keithley 2636B (channel A and B)":refnum<visa-resource-name>="GPIB0::26::INSTR"
  in  "stop":bool
  out "Time (s)":dbl=4994.9
  in  "Folder":path=path "D:/Pranava/Data/STS/MA2479"
  out "data":dbl[](array[numeric])=[4994.9, -0.0020110788365, 8.848779425879616e-11, 2.798241597479316e-06, 3.162264271194698e-05, -1.6999999999999718, -4.2499999999999295e-08]
  out "File path 1":path=path "D:/Pranava/Data/STS/MA2479/003_MA2479_[Dev110]_40uV_50pA_17.7777Hz_4thorder_300ms_0T_measureX_float_20xaverage.dat"
  # ".dat"
  # "Set Voltage sweep Device 1 (V)"
  # ".dat"
  # "Set Voltage sweep Device 2 (V)"
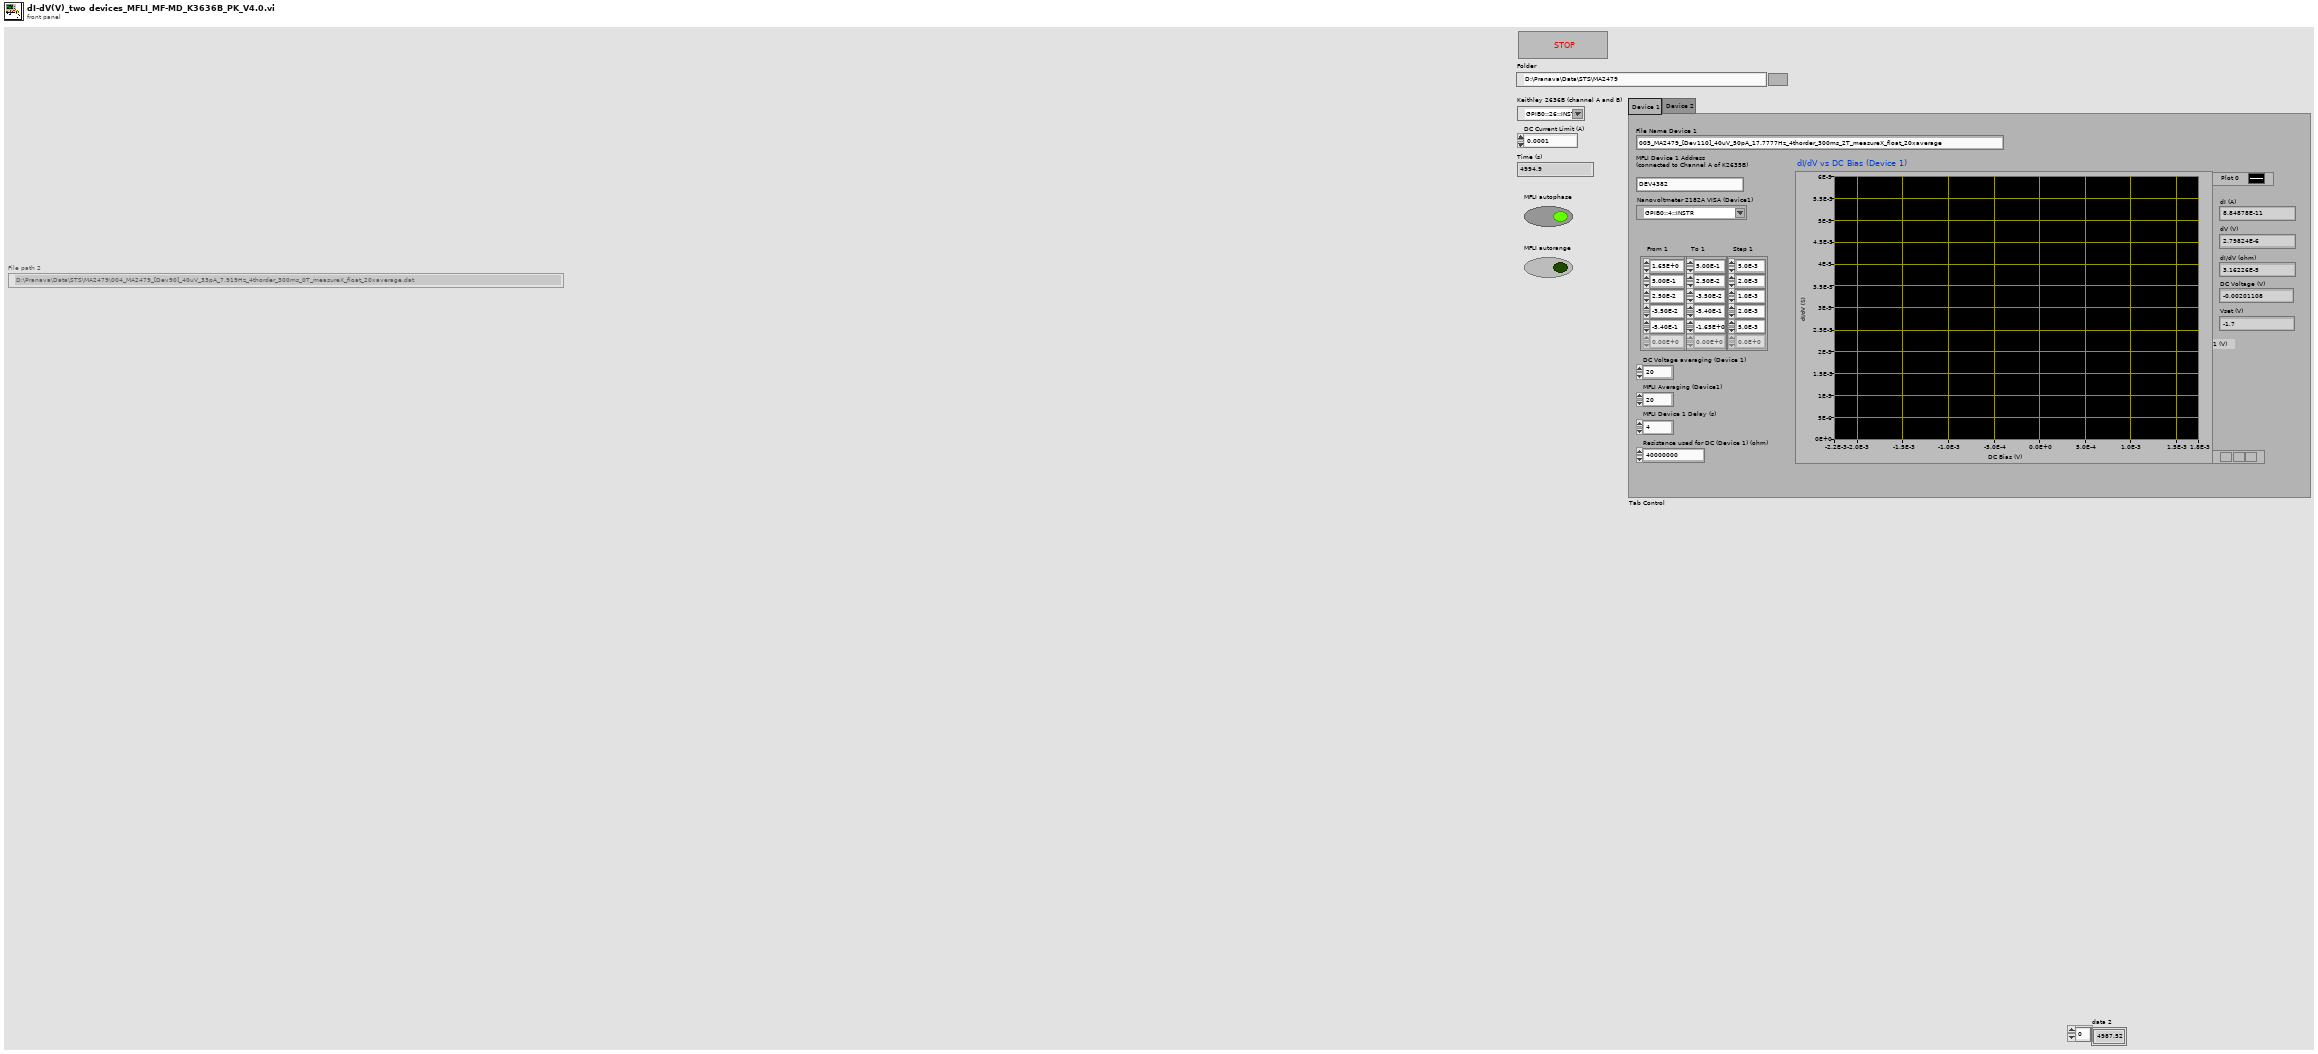
[diagram p1: front panel]
types:
  T1 = enum16{"open", "replace", "create", "open or create", "replace or create", "replace or create with confirmation"}
  T2 = typedef "Zurich Instruments LabOne.lvlib/ziTypeHandle.ctl" = cluster{"handleValid":bool, "Conn":u64, "Path Prefix":string, "Handle":u64, "Connected":bool, "Clockbase(s)":dbl}
  T3 = typedef "Zurich Instruments LabOne.lvlib/ziTypeDemodSampleSingle.ctl" = cluster{"Timestamps (ticks)":u64, "X (Vrms)":dbl, "Y (Vrms)":dbl, "Osc Phase (deg)":dbl, "Freq (Hz)":dbl, "DIO":u32, "AuxIn0 (V)":dbl, "AuxIn1 (V)":dbl, "Trigger":u32}
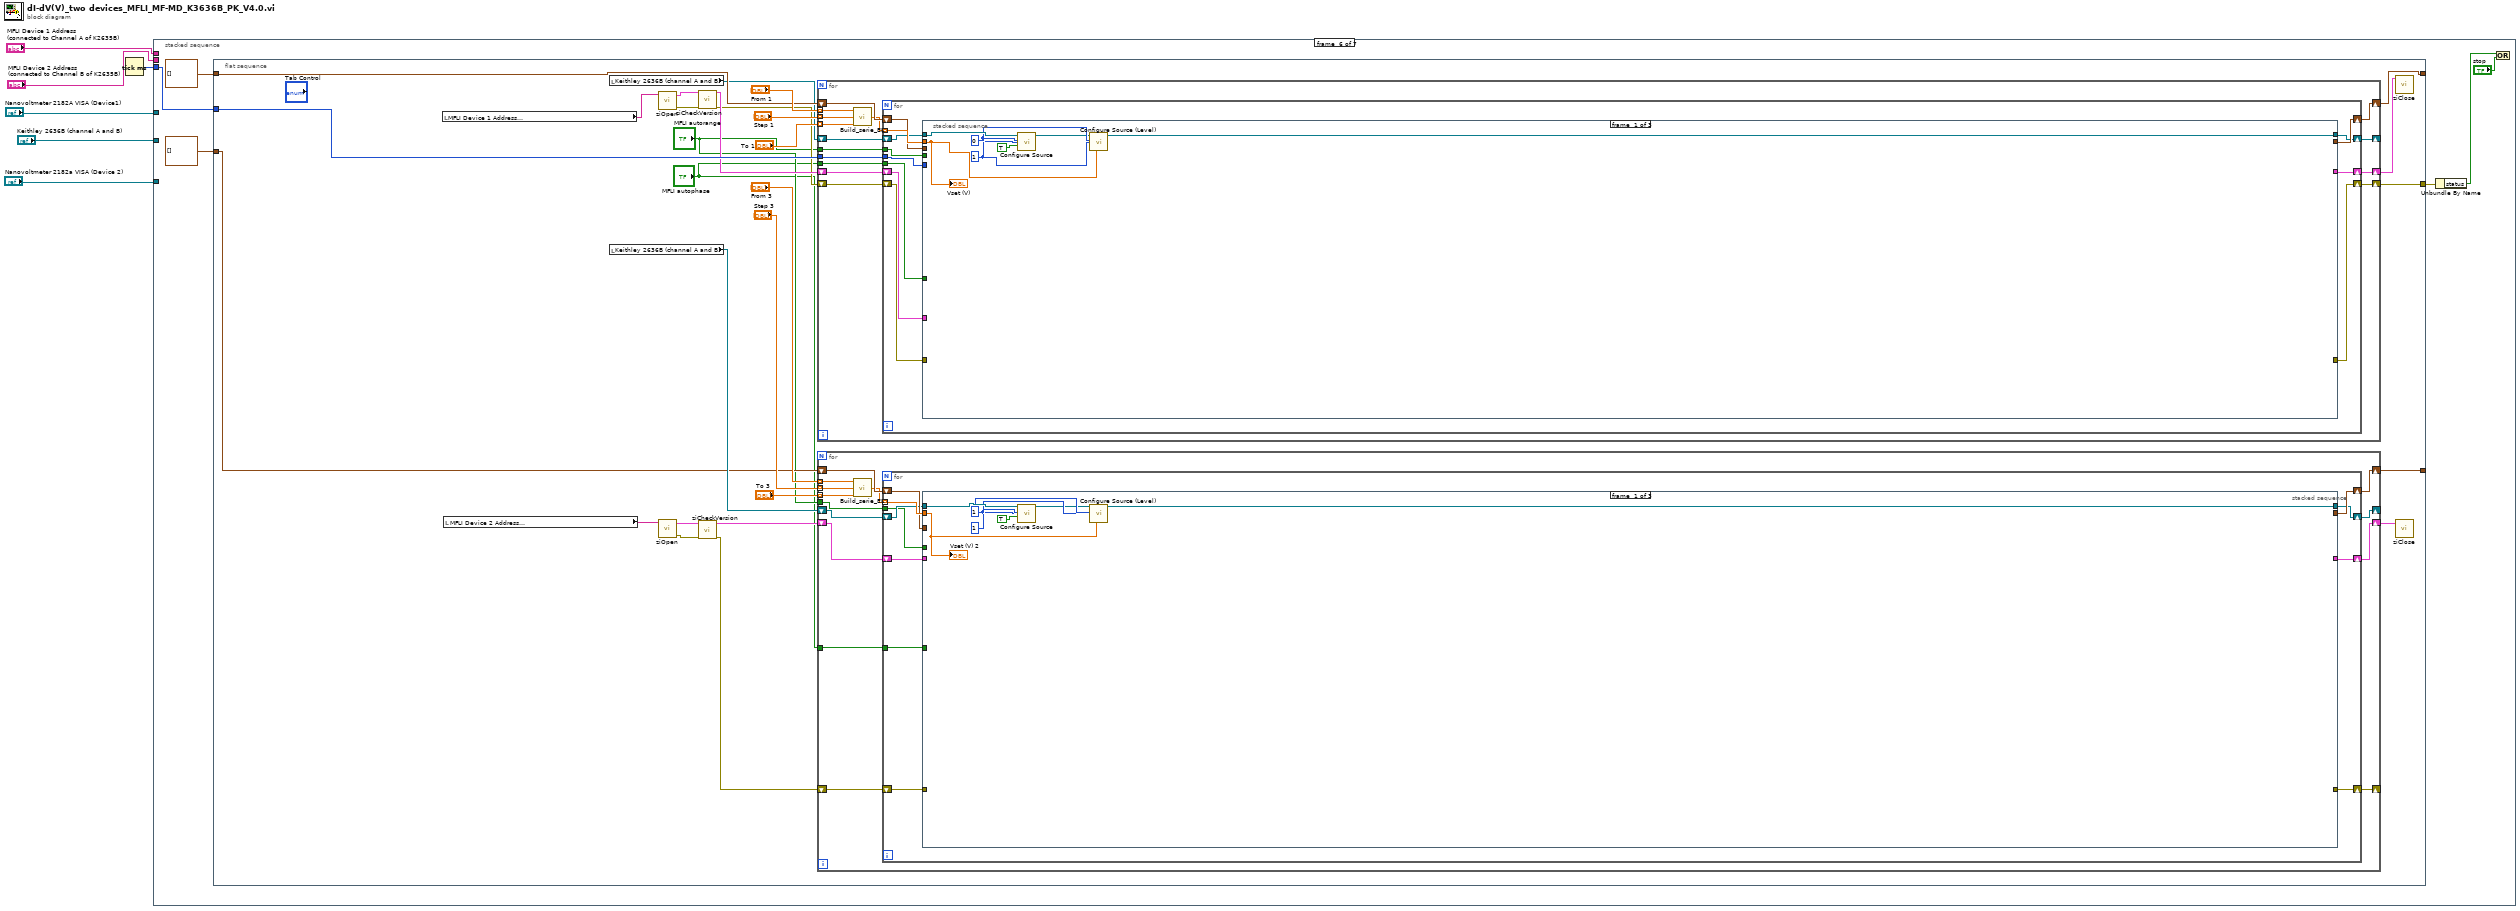
[diagram p0: block diagram]
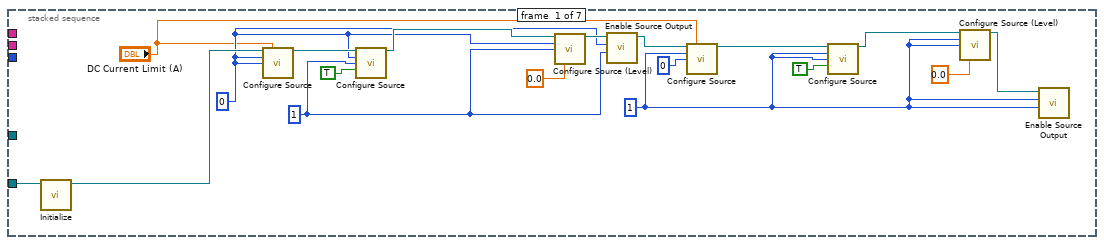
[diagram p2: hidden frame]
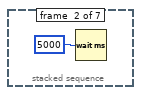
[diagram p3: hidden frame]
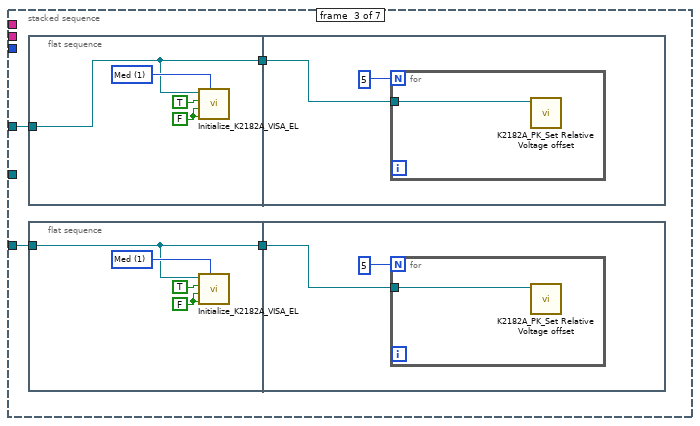
[diagram p4: hidden frame]
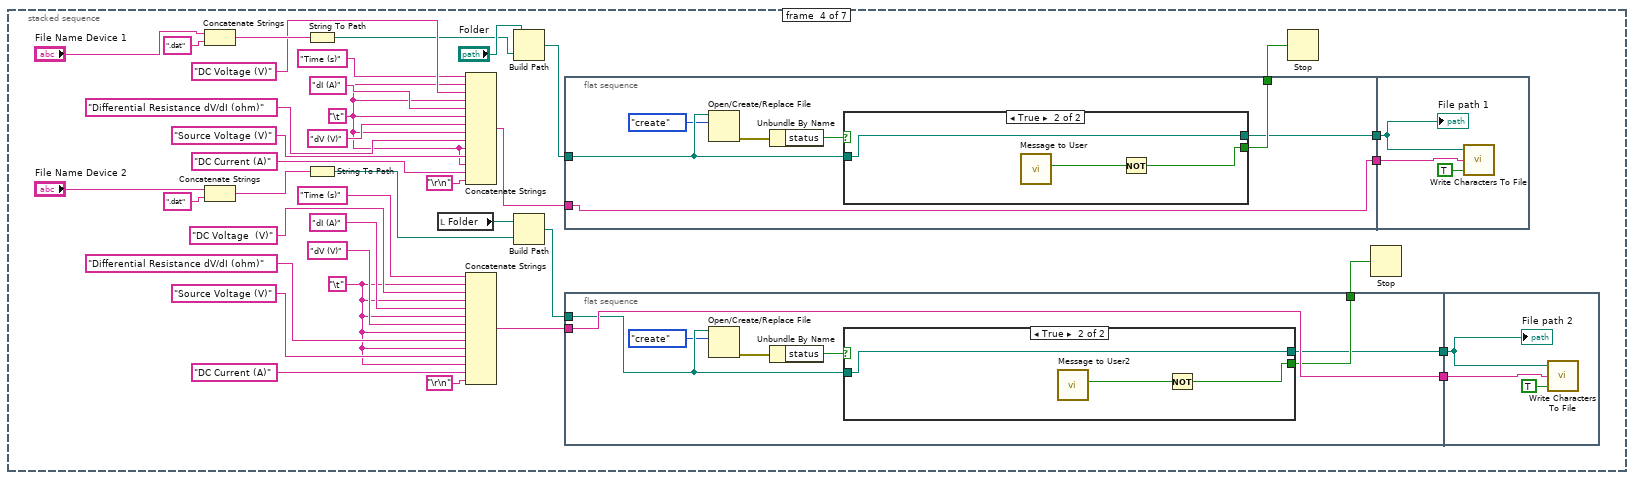
[diagram p5: hidden frame]
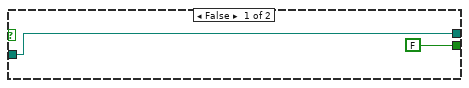
[diagram p6: hidden frame]
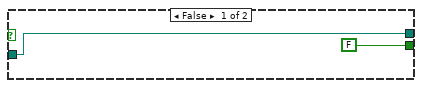
[diagram p7: hidden frame]
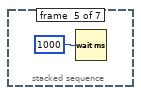
[diagram p8: hidden frame]
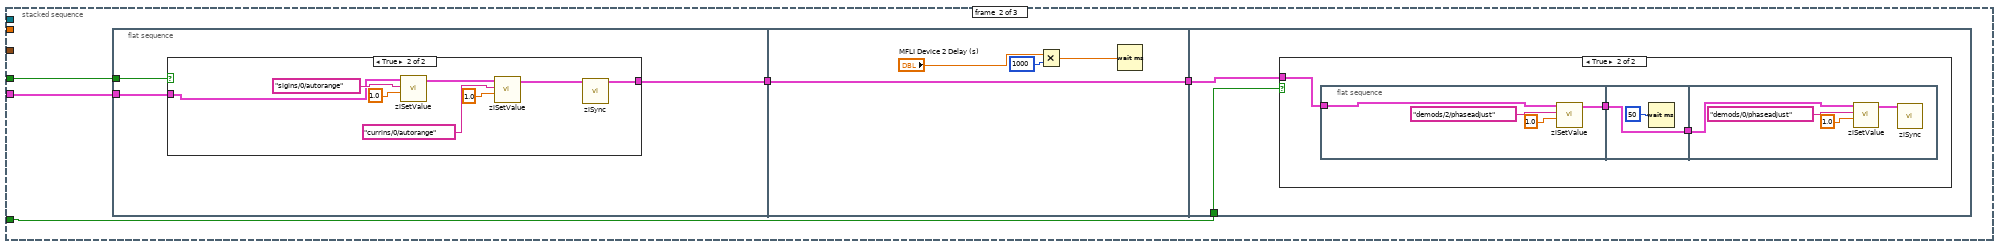
[diagram p9: hidden frame]
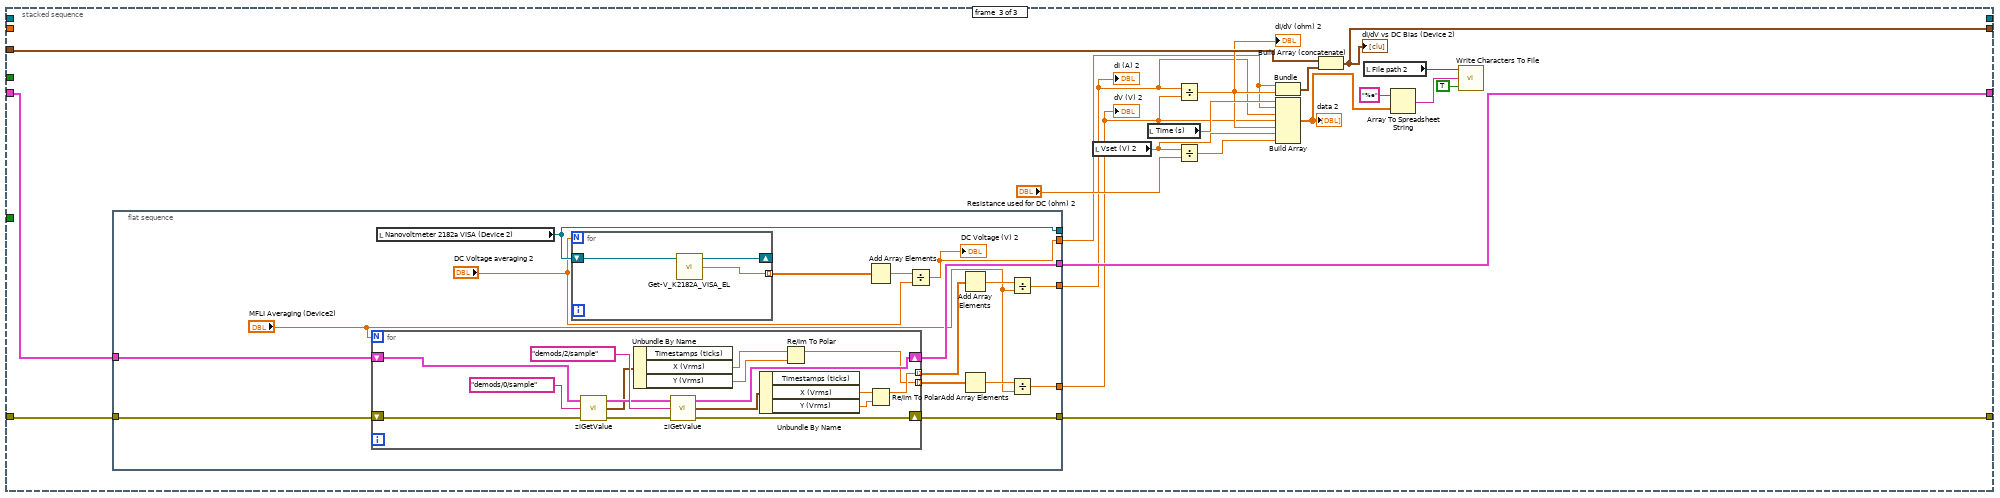
[diagram p12: hidden frame]
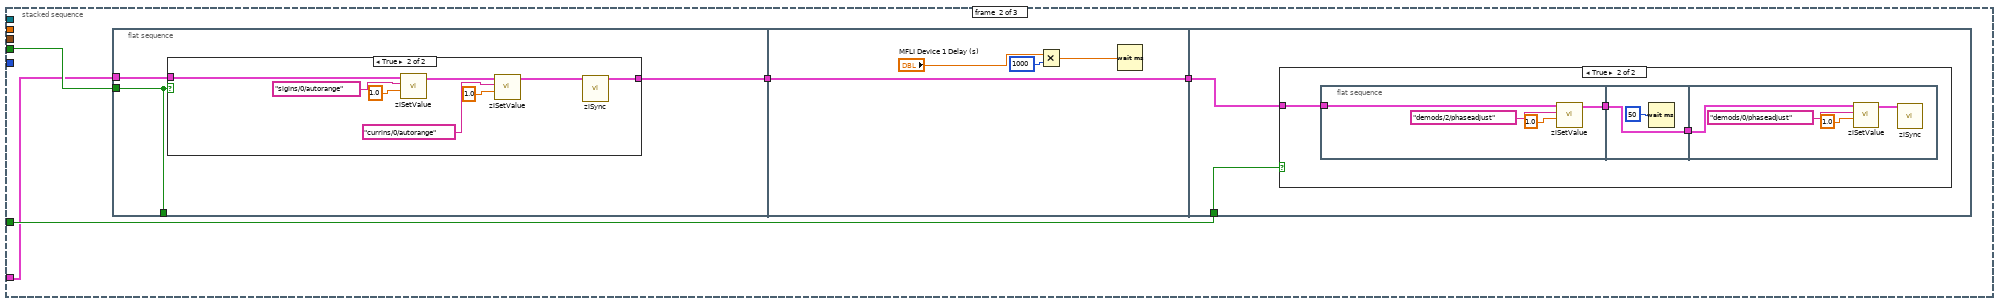
[diagram p13: hidden frame]
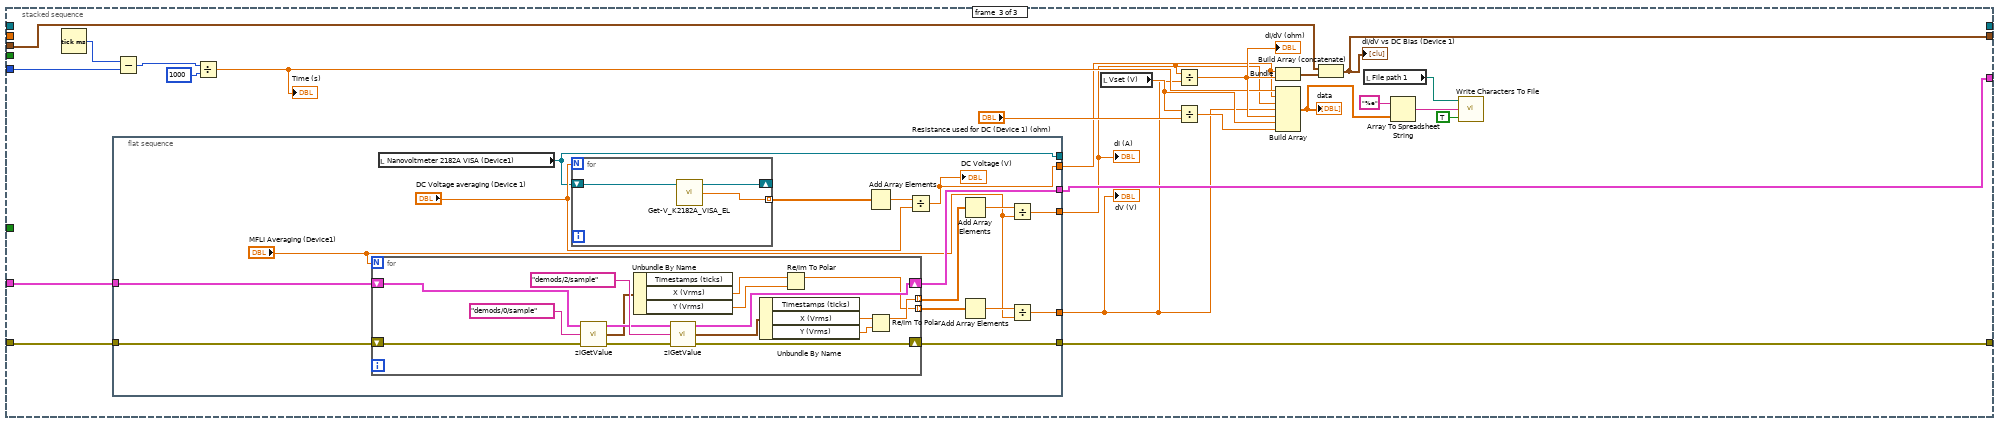
[diagram p16: hidden frame]
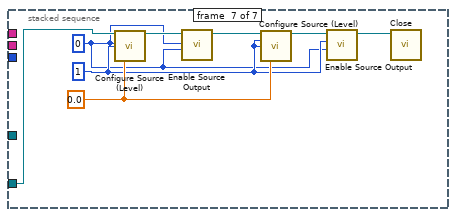
[diagram p17: hidden frame]
diagram:
  n1 = Tick Count (ms)() -> (millisecond timer value=w4:u32)
  n2 = stacked-sequence {
    tunnel: "Nanovoltmeter 2182A VISA (Device1)" -> [_ _ w29 _ _ _ _]
    tunnel: "MFLI Device 1 Address\n(connected to Channel A of K2635B)" -> [_ _ _ _ _ _ _]
    tunnel: w4 -> [_ _ _ _ _ w117 _]
    tunnel: "Keithley 2636B (channel A and B)" -> [w24 _ _ _ _ _ w405]
    tunnel: "Nanovoltmeter 2182a VISA (Device 2)" -> [_ _ w26 _ _ _ _]
    tunnel: "MFLI Device 2 Address\n(connected to Channel B of K2635B)" -> [_ _ _ _ _ _ _]
    frame #0 {
      w7 = 1
      w18 = 0
      w16 = 1
      n3 = call <instrlib>:"Initialize.vi"("VISA resource name"=w24) -> ("VISA resource name out"=w23:refnum<visa-resource-name>)  [unwired: 9 in, 1 out]
      n4 = call-poly <instrlib>:"Configure Source.vi"("VISA resource name"=w23, "Current Limit (0.1 A)"="DC Current Limit (A)", "Source Measure Unit Channel (0: Channel A)"=w18, "Limit Type (1: Voltage)"=w18) -> ("VISA resource name out"=w22:refnum<visa-resource-name>)  [unwired: 10 in, 1 out]
      n5 = call-poly <instrlib>:"Configure Source.vi"("VISA resource name"=w22, "Source Measure Unit Channel (0: Channel A)"=w18, "Range Type (1: Voltage)"=w16, "Auto Range (T: Enable)"=TRUE) -> ("VISA resource name out"=w21:refnum<visa-resource-name>)  [unwired: 10 in, 1 out]
      n6 = call <instrlib>:"Configure Source (Level).vi"("VISA resource name"=w21, "Source Measure Unit Channel (0: Channel A)"=w18, "Level Type (1: Voltage)"=w16, "Voltage Level (0 V)"=0.0) -> ("VISA resource name out"=w20:refnum<visa-resource-name>)  [unwired: 10 in, 1 out]
      n7 = call <instrlib>:"Enable Source Output.vi"("Output Mode (0: Turn off)"=w16, "Source Measure Unit Channel (0: Channel A)"=w18, "VISA resource name"=w20) -> ("VISA resource name out"=w10:refnum<visa-resource-name>)  [unwired: 7 in, 1 out]
      n8 = call-poly <instrlib>:"Configure Source.vi"("VISA resource name"=w10, "Current Limit (0.1 A)"="DC Current Limit (A)", "Source Measure Unit Channel (0: Channel A)"=w7, "Limit Type (1: Voltage)"=0) -> ("VISA resource name out"=w15:refnum<visa-resource-name>)  [unwired: 10 in, 1 out]
      n9 = call-poly <instrlib>:"Configure Source.vi"("VISA resource name"=w15, "Source Measure Unit Channel (0: Channel A)"=w7, "Range Type (1: Voltage)"=w7, "Auto Range (T: Enable)"=TRUE) -> ("VISA resource name out"=w14:refnum<visa-resource-name>)  [unwired: 10 in, 1 out]
      n10 = call <instrlib>:"Configure Source (Level).vi"("VISA resource name"=w14, "Source Measure Unit Channel (0: Channel A)"=w7, "Level Type (1: Voltage)"=w7, "Voltage Level (0 V)"=0.0) -> ("VISA resource name out"=w13:refnum<visa-resource-name>)  [unwired: 10 in, 1 out]
      n11 = call <instrlib>:"Enable Source Output.vi"("Output Mode (0: Turn off)"=w7, "Source Measure Unit Channel (0: Channel A)"=w7, "VISA resource name"=w13) -> ()  [unwired: 7 in, 2 out]
    }
    frame #1 {
      n12 = Wait (ms)(milliseconds to wait=5000) -> ()  [unwired: 1 out]
    }
    frame #2 {
      n13 = flat-sequence {
        tunnel: w29 -> [w37]
        tunnel: [w37] -> w28
        tunnel: w28 -> [w41]
        frame #0 {
          w39 = u16 1 items=["Slow", "Med", "Fast"] ("Rate (NPLC)")
          w40 = FALSE ("Auto range?")
          n14 = call "Initialize_K2182A_VISA_EL.vi"("VISA address"=w37, "Auto range?"=TRUE, "Analog LPass\nFilter?"=w40, "DC\nFilter?"=w40, "Rate (NPLC)"=w39) -> ()  [unwired: 1 in, 1 out]
        }
        frame #1 {
          n15 = for {
            N: 5 ("Numeric") -> [_]
            tunnel: w41 -> [w43]
            n16 = call "K2182A_PK_Set Relative Voltage offset.vi"("VISA address"=w43) -> ()  [unwired: 11 in]
          }
        }
      }
      n17 = flat-sequence {
        tunnel: w26 -> [w30]
        tunnel: [w30] -> w27
        tunnel: w27 -> [w34]
        frame #0 {
          w32 = u16 1 items=["Slow", "Med", "Fast"] ("Rate (NPLC)")
          w33 = FALSE ("Auto range?")
          n18 = call "Initialize_K2182A_VISA_EL.vi"("VISA address"=w30, "Auto range?"=TRUE, "Analog LPass\nFilter?"=w33, "DC\nFilter?"=w33, "Rate (NPLC)"=w32) -> ()  [unwired: 1 in, 1 out]
        }
        frame #1 {
          n19 = for {
            N: 5 ("Numeric") -> [_]
            tunnel: w34 -> [w36]
            n20 = call "K2182A_PK_Set Relative Voltage offset.vi"("VISA address"=w36) -> ()  [unwired: 11 in]
          }
        }
      }
    }
    frame #3 {
      w47 = "\t"
      w64 = "\t"
      n21 = Concatenate Strings("File Name Device 1", ".dat" ("string")) -> (w78:string)
      n22 = Concatenate Strings("File Name Device 2", ".dat" ("string")) -> (w59:string)
      n23 = String To Path(string=w78) -> (path=w70:path)
      n24 = String To Path(string=w59) -> (path=w53:path)
      n25 = local read "Folder"() -> (w45:path)
      n26 = Concatenate Strings("Time (s)", w64, "DC Voltage (V)" ("string"), w64, "dI (A)" ("string"), w64, "dV (V)" ("string"), w64, "Differential Resistance dV/dI (ohm)", w64, "Source Voltage (V)", w64, "DC Current (A)", "\r\n") -> (w79:string)
      n27 = Concatenate Strings("Time (s)", w47, "DC Voltage  (V)" ("string"), w47, "dI (A)" ("string"), w47, "dV (V)" ("string"), w47, "Differential Resistance dV/dI (ohm)", w47, "Source Voltage (V)", w47, "DC Current (A)", "\r\n") -> (w60:string)
      n28 = Build Path(base path="Folder", name or relative path=w70) -> (appended path=w69:path)
      n29 = Build Path(base path=w45, name or relative path=w53) -> (appended path=w52:path)
      n30 = flat-sequence {
        tunnel: w69 -> [w100]
        tunnel: w79 -> [w103]
        tunnel: [w103] -> w81
        tunnel: [w102] -> w76
        tunnel: [w101] -> w80
        tunnel: w81 -> [w110]
        tunnel: w80 -> [w109]
        frame #0 {
          n31 = Open/Create/Replace File(file path (use dialog)=w100, operation (0:open)=T1."create") -> (error out=w99:errorcluster)  [unwired: 4 in, 2 out]
          n32 = Unbundle By Name(w99) -> ("status"=w97:bool)
          n33 = case shown="True" w97 {
            tunnel: [FALSE ("Yes") w107] -> w102
            tunnel: [w104 w106] -> w101
            tunnel: w100 -> [w104 w106]
            frame False {
            }
            frame True {
              n34 = call "Message to User"() -> ("Yes"=w108:bool)  [unwired: 10 in, 1 out]
              n35 = Not(x=w108) -> (.not. x?=w107:bool)
            }
          }
        }
        frame #1 {
          n36 = call <vilib>:"Write Characters To File.vi"("append to file? (new file:F)"=TRUE, "character string"=w110, "file path (dialog if empty)"=w109) -> ()  [unwired: 2 in, 1 out]
          "File path 1" <- w109
        }
      }
      n37 = flat-sequence {
        tunnel: w52 -> [w85]
        tunnel: w60 -> [w88]
        tunnel: [w88] -> w62
        tunnel: [w87] -> w58
        tunnel: [w86] -> w61
        tunnel: w62 -> [w95]
        tunnel: w61 -> [w94]
        frame #0 {
          n38 = Open/Create/Replace File(file path (use dialog)=w85, operation (0:open)=T1."create") -> (error out=w84:errorcluster)  [unwired: 4 in, 2 out]
          n39 = Unbundle By Name(w84) -> ("status"=w82:bool)
          n40 = case shown="True" w82 {
            tunnel: [FALSE ("Yes") w92] -> w87
            tunnel: [w89 w91] -> w86
            tunnel: w85 -> [w89 w91]
            frame False {
            }
            frame True {
              n41 = call "Message to User2"() -> ("Yes"=w93:bool)  [unwired: 10 in, 1 out]
              n42 = Not(x=w93) -> (.not. x?=w92:bool)
            }
          }
        }
        frame #1 {
          n43 = call <vilib>:"Write Characters To File.vi"("append to file? (new file:F)"=TRUE, "character string"=w95, "file path (dialog if empty)"=w94) -> ()  [unwired: 2 in, 1 out]
          "File path 2" <- w94
        }
      }
      n44 = Stop(stop? (T)=w76) -> ()
      n45 = Stop(stop? (T)=w58) -> ()
    }
    frame #4 {
      n46 = Wait (ms)(milliseconds to wait=u32 1000) -> ()  [unwired: 1 out]
    }
    frame #5 {
      n47 = flat-sequence {
        tunnel: [w141] -> w115
        tunnel: [w140] -> _
        tunnel: [w125] -> _
        tunnel: cluster{dbl, "Field Reading":dbl}[] [] -> [w121]
        tunnel: cluster{dbl, "Field Reading":dbl}[] [] -> [w143]
        tunnel: w117 -> [w142]
        frame #0 {
          n48 = local read "MFLI Device 1 Address\n(connected to Channel A of K2635B)"() -> (w137:string)
          n49 = local read "MFLI Device 2 Address\n(connected to Channel B of K2635B)"() -> (w130:string)
          n50 = local read "Keithley 2636B (channel A and B)"() -> (w133:refnum<visa-resource-name>)
          n51 = local read "Keithley 2636B (channel A and B)"() -> (w126:refnum<visa-resource-name>)
          n52 = call <instrlib>:"ziOpen.vi"("Address"=w137) -> ("Error Out"=w136:errorcluster, "HandleOut"=w139:T2)  [unwired: 3 in, 1 out]
          n53 = call <instrlib>:"ziOpen.vi"("Address"=w130) -> ("Error Out"=w129:errorcluster, "HandleOut"=w132:T2)  [unwired: 3 in, 1 out]
          n54 = call <instrlib>:"ziCheckVersion.vi"("Handle In"=w139, "Error In"=w136) -> ("Handle Out"=w138:T2, "Error Out"=w135:errorcluster)  [unwired: 11 in, 1 out]
          n55 = call <instrlib>:"ziCheckVersion.vi"("Handle In"=w132, "Error In"=w129) -> ("Handle Out"=w131:T2, "Error Out"=w128:errorcluster)  [unwired: 11 in, 1 out]
          n56 = for {
            tunnel: "From 1" -> [w281] mode=indexing
            tunnel: "To 1" -> [w280] mode=indexing
            tunnel: "Step 1" -> [w279] mode=indexing
            shift-right: [w283] -> w140
            shift-left: w143 -> [w284]
            tunnel: w142 -> [w278]
            shift-right: [w276] -> w134
            shift-left: w138 -> [w277]
            shift-right: [w275] -> w141
            shift-left: w135 -> [w274]
            shift-right: [w272] -> _
            shift-left: w133 -> [w273]
            tunnel: "MFLI autorange" -> [w271]
            tunnel: "MFLI autophase" -> [w270]
            n57 = call "Build_serie_EL.vi"("end value"=w280, "increment"=w279, "start value"=w281) -> ("output array"=w282:dbl[])
            n58 = for {
              tunnel: w282 -> [w296] mode=indexing
              shift-right: [w294] -> w283
              shift-left: w284 -> [w295]
              tunnel: w278 -> [w293]
              shift-right: [w291] -> w276
              shift-left: w277 -> [w292]
              shift-right: [w290] -> w275
              shift-left: w274 -> [w289]
              shift-right: [w287] -> w272
              shift-left: w273 -> [w288]
              tunnel: w271 -> [w286]
              tunnel: w270 -> [w285]
              n59 = stacked-sequence {
                tunnel: w295 -> [_ _ w362]
                tunnel: w296 -> [w303 _ _]
                tunnel: [_ _ w361] -> w294
                tunnel: w293 -> [_ _ w358]
                tunnel: w292 -> [_ w304 w354]
                tunnel: [_ _ w353] -> w291
                tunnel: [_ _ w352] -> w290
                tunnel: w289 -> [_ _ w351]
                tunnel: w288 -> [w301 _ _]
                tunnel: [w302 _ _] -> w287
                tunnel: w286 -> [_ w306 _]
                tunnel: w285 -> [_ w305 _]
                frame #0 {
                  w300 = 0
                  w299 = 1
                  n60 = call-poly <instrlib>:"Configure Source.vi"("VISA resource name"=w301, "Source Measure Unit Channel (0: Channel A)"=w300, "Range Type (1: Voltage)"=w299, "Auto Range (T: Enable)"=TRUE) -> ("VISA resource name out"=w297:refnum<visa-resource-name>)  [unwired: 10 in, 1 out]
                  n61 = call <instrlib>:"Configure Source (Level).vi"("VISA resource name"=w297, "Source Measure Unit Channel (0: Channel A)"=w300, "Level Type (1: Voltage)"=w299, "Voltage Level (0 V)"=w303) -> ("VISA resource name out"=w302:refnum<visa-resource-name>)  [unwired: 10 in, 1 out]
                  "Vset (V)" <- w303
                }
                frame #1 {
                  n62 = flat-sequence {
                    tunnel: [w309] -> _
                    tunnel: w304 -> [w311]
                    tunnel: [w310] -> w308
                    tunnel: w306 -> [w309]
                    tunnel: [w321] -> w307
                    tunnel: w308 -> [w321]
                    tunnel: w307 -> [w326]
                    tunnel: w305 -> [w325]
                    frame #0 {
                      n63 = case shown="True" w309 {
                        tunnel: w311 -> [w312 w314]
                        tunnel: [w312 w313] -> w310
                        frame False {
                        }
                        frame True {
                          n64 = call-poly <instrlib>:"ziSetValue.vi"("Value"=1.0, "Path"="sigins/0/autorange", "Handle In"=w314) -> ("Handle Out"=w319:T2)  [unwired: 2 in, 1 out]
                          n65 = call-poly <instrlib>:"ziSetValue.vi"("Value"=1.0, "Path"="currins/0/autorange", "Handle In"=w319) -> ("Handle Out"=w320:T2)  [unwired: 2 in, 1 out]
                          n66 = call <instrlib>:"ziSync.vi"("Handle In"=w320) -> ("Handle Out"=w313:T2)  [unwired: 13 in, 1 out]
                        }
                      }
                    }
                    frame #1 {
                      n67 = Multiply(x="MFLI Device 1 Delay (s)", y=1000) -> (x*y=w324:dbl)
                      n68 = Wait (ms)(milliseconds to wait=w324) -> ()  [unwired: 1 out]
                    }
                    frame #2 {
                      n69 = case shown="True" w325 {
                        tunnel: w326 -> [_ w327]
                        frame False {
                        }
                        frame True {
                          n70 = flat-sequence {
                            tunnel: [w333] -> w329
                            tunnel: w327 -> [w330]
                            tunnel: w329 -> [w335]
                            tunnel: [w335] -> w328
                            tunnel: w328 -> [w336]
                            frame #0 {
                              n71 = call-poly <instrlib>:"ziSetValue.vi"("Value"=1.0, "Path"="demods/2/phaseadjust", "Handle In"=w330) -> ("Handle Out"=w333:T2)  [unwired: 2 in, 1 out]
                            }
                            frame #1 {
                              n72 = Wait (ms)(milliseconds to wait=50) -> ()  [unwired: 1 out]
                            }
                            frame #2 {
                              n73 = call-poly <instrlib>:"ziSetValue.vi"("Value"=1.0, "Path"="demods/0/phaseadjust", "Handle In"=w336) -> ("Handle Out"=w337:T2)  [unwired: 2 in, 1 out]
                              n74 = call <instrlib>:"ziSync.vi"("Handle In"=w337) -> ()  [unwired: 13 in, 2 out]
                            }
                          }
                        }
                      }
                    }
                  }
                }
                frame #2 {
                  n75 = Tick Count (ms)() -> (millisecond timer value=w359:u32)
                  n76 = flat-sequence {
                    tunnel: [w369] -> w342
                    tunnel: [w367] -> w341
                    tunnel: [w378] -> w352
                    tunnel: [w379] -> w353
                    tunnel: [w374] -> _
                    tunnel: w351 -> [w372]
                    tunnel: w354 -> [w373]
                    tunnel: [w364] -> w340
                    frame #0 {
                      n77 = for {
                        N: "MFLI Averaging (Device1)" -> [_]
                        tunnel: [w393] -> w366 mode=indexing
                        tunnel: [w392] -> w368 mode=indexing
                        shift-right: [w395] -> w379
                        shift-left: w373 -> [w381]
                        shift-right: [w394] -> w378
                        shift-left: w372 -> [w380]
                        n78 = call-poly <instrlib>:"ziGetValue.vi"("error in"=w380, "Path"="demods/0/sample", "Handle In"=w381) -> ("error out"=w386:errorcluster, "Demod Sample Out"=w384:T3, "Handle Out"=w387:T2)
                        n79 = Unbundle By Name(w384) -> ("X (Vrms)"=w383:dbl, "Y (Vrms)"=w382:dbl)  [unwired: 1 out]
                        n80 = call-poly <instrlib>:"ziGetValue.vi"("error in"=w386, "Path"="demods/2/sample", "Handle In"=w387) -> ("error out"=w394:errorcluster, "Demod Sample Out"=w390:T3, "Handle Out"=w395:T2)
                        n81 = Unbundle By Name(w390) -> ("X (Vrms)"=w389:dbl, "Y (Vrms)"=w388:dbl)  [unwired: 1 out]
                        n82 = Re/Im To Polar(2:w382, 3:w383) -> (1:w392:dbl)  [unwired: 1 out]
                        n83 = Re/Im To Polar(2:w388, 3:w389) -> (1:w393:dbl)  [unwired: 1 out]
                      }
                      n84 = local read "Nanovoltmeter 2182A VISA (Device1)"() -> (w374:refnum<visa-resource-name>)
                      n85 = for {
                        N: "DC Voltage averaging (Device 1)" -> [_]
                        tunnel: [w397] -> w376 mode=indexing
                        shift-right: [w396] -> _
                        shift-left: w374 -> [w398]
                        n86 = call "Get-V_K2182A_VISA_EL.vi"("VISA K2182A"=w398) -> ("V (V)"=w397:dbl, "VISA K2182A out"=w396:refnum<visa-resource-name>)  [unwired: 2 in, 1 out]
                      }
                      n87 = Add Array Elements(numeric array=w376) -> (sum=w377:dbl)
                      n88 = Divide(x=w377, y="DC Voltage averaging (Device 1)") -> (x/y=w364:dbl)
                      "DC Voltage (V)" <- w364
                      n89 = Add Array Elements(numeric array=w366) -> (sum=w371:dbl)
                      n90 = Add Array Elements(numeric array=w368) -> (sum=w370:dbl)
                      n91 = Divide(x=w371, y="MFLI Averaging (Device1)") -> (x/y=w367:dbl)
                      n92 = Divide(x=w370, y="MFLI Averaging (Device1)") -> (x/y=w369:dbl)
                    }
                  }
                  n93 = Subtract(x=w359, y=w358) -> (x-y=w357:u32)
                  n94 = Divide(x=w357, y=1000) -> (x/y=w355:dbl)
                  "Time (s)" <- w355
                  n95 = local read "Vset (V)"() -> (w344:dbl)
                  n96 = Divide(x=w341, y=w342) -> (x/y=w360:dbl)
                  "dI/dV (ohm)" <- w360
                  n97 = Divide(x=w344, y="Resistance used for DC (Device 1) (ohm)") -> (x/y=w343:dbl)
                  n98 = Bundle(w340, w360) -> (w363:cluster{dbl, dbl})  [unwired: 1 in]
                  n99 = Build Array(w355, w340, w341, w342, w360, w344, w343) -> (w346:dbl[])
                  "data" <- w346
                  n100 = Build Array (concatenate)(w362, w363) -> (w361:cluster{dbl, "Field Reading":dbl}[])
                  "dI/dV vs DC Bias (Device 1)" <- w361
                  n101 = local read "File path 1"() -> (w348:path)
                  n102 = Array To Spreadsheet String(array=w346, 3:"%e" ("format string")) -> (spreadsheet string=w349:string)  [unwired: 1 in]
                  n103 = call <vilib>:"Write Characters To File.vi"("append to file? (new file:F)"=TRUE, "character string"=w349, "file path (dialog if empty)"=w348) -> ()  [unwired: 2 in, 1 out]
                  "dI (A)" <- w341
                  "dV (V)" <- w342
                }
              }
            }
          }
          n104 = for {
            tunnel: "From 3" -> [w157] mode=indexing
            tunnel: "To 3" -> [w156] mode=indexing
            tunnel: "Step 3" -> [w155] mode=indexing
            shift-right: [w159] -> w125
            shift-left: w121 -> [w160]
            shift-right: [w153] -> w127
            shift-left: w131 -> [w154]
            shift-right: [w152] -> _
            shift-left: w128 -> [w151]
            shift-right: [w149] -> _
            shift-left: w126 -> [w150]
            tunnel: "MFLI autophase" -> [w148]
            tunnel: "MFLI autorange" -> [w147]
            n105 = call "Build_serie_EL.vi"("end value"=w156, "increment"=w155, "start value"=w157) -> ("output array"=w158:dbl[])
            n106 = for {
              tunnel: w158 -> [w171] mode=indexing
              shift-right: [w169] -> w159
              shift-left: w160 -> [w170]
              shift-right: [w167] -> w153
              shift-left: w154 -> [w168]
              shift-right: [w166] -> w152
              shift-left: w151 -> [w165]
              shift-right: [w163] -> w149
              shift-left: w150 -> [w164]
              tunnel: w148 -> [w162]
              tunnel: w147 -> [w161]
              n107 = stacked-sequence {
                tunnel: w170 -> [_ _ w233]
                tunnel: w171 -> [w172 _ _]
                tunnel: [_ _ w218] -> w169
                tunnel: w168 -> [_ w181 w232]
                tunnel: [_ _ w231] -> w167
                tunnel: [_ _ w230] -> w166
                tunnel: w165 -> [_ _ w229]
                tunnel: w164 -> [w177 _ _]
                tunnel: [w178 _ _] -> w163
                tunnel: w162 -> [_ w183 _]
                tunnel: w161 -> [_ w182 _]
                frame #0 {
                  w176 = 1
                  w175 = 1
                  n108 = call-poly <instrlib>:"Configure Source.vi"("VISA resource name"=w177, "Source Measure Unit Channel (0: Channel A)"=w176, "Range Type (1: Voltage)"=w175, "Auto Range (T: Enable)"=TRUE) -> ("VISA resource name out"=w173:refnum<visa-resource-name>)  [unwired: 10 in, 1 out]
                  n109 = call <instrlib>:"Configure Source (Level).vi"("VISA resource name"=w173, "Source Measure Unit Channel (0: Channel A)"=w176, "Level Type (1: Voltage)"=w175, "Voltage Level (0 V)"=w172) -> ("VISA resource name out"=w178:refnum<visa-resource-name>)  [unwired: 10 in, 1 out]
                  "Vset (V) 2" <- w172
                }
                frame #1 {
                  n110 = flat-sequence {
                    tunnel: w182 -> [w186]
                    tunnel: w181 -> [w185]
                    tunnel: [w184] -> w179
                    tunnel: [w196] -> w180
                    tunnel: w179 -> [w196]
                    tunnel: w183 -> [w201]
                    tunnel: w180 -> [w200]
                    frame #0 {
                      n111 = case shown="True" w186 {
                        tunnel: w185 -> [w187 w189]
                        tunnel: [w187 w188] -> w184
                        frame False {
                        }
                        frame True {
                          n112 = call-poly <instrlib>:"ziSetValue.vi"("Value"=1.0, "Path"="sigins/0/autorange", "Handle In"=w189) -> ("Handle Out"=w194:T2)  [unwired: 2 in, 1 out]
                          n113 = call-poly <instrlib>:"ziSetValue.vi"("Value"=1.0, "Path"="currins/0/autorange", "Handle In"=w194) -> ("Handle Out"=w195:T2)  [unwired: 2 in, 1 out]
                          n114 = call <instrlib>:"ziSync.vi"("Handle In"=w195) -> ("Handle Out"=w188:T2)  [unwired: 13 in, 1 out]
                        }
                      }
                    }
                    frame #1 {
                      n115 = Multiply(x="MFLI Device 2 Delay (s)", y=1000) -> (x*y=w199:dbl)
                      n116 = Wait (ms)(milliseconds to wait=w199) -> ()  [unwired: 1 out]
                    }
                    frame #2 {
                      n117 = case shown="True" w201 {
                        tunnel: w200 -> [_ w202]
                        frame False {
                        }
                        frame True {
                          n118 = flat-sequence {
                            tunnel: [w208] -> w204
                            tunnel: w202 -> [w205]
                            tunnel: w204 -> [w210]
                            tunnel: [w210] -> w203
                            tunnel: w203 -> [w211]
                            frame #0 {
                              n119 = call-poly <instrlib>:"ziSetValue.vi"("Value"=1.0, "Path"="demods/2/phaseadjust", "Handle In"=w205) -> ("Handle Out"=w208:T2)  [unwired: 2 in, 1 out]
                            }
                            frame #1 {
                              n120 = Wait (ms)(milliseconds to wait=50) -> ()  [unwired: 1 out]
                            }
                            frame #2 {
                              n121 = call-poly <instrlib>:"ziSetValue.vi"("Value"=1.0, "Path"="demods/0/phaseadjust", "Handle In"=w211) -> ("Handle Out"=w212:T2)  [unwired: 2 in, 1 out]
                              n122 = call <instrlib>:"ziSync.vi"("Handle In"=w212) -> ()  [unwired: 13 in, 2 out]
                            }
                          }
                        }
                      }
                    }
                  }
                }
                frame #2 {
                  n123 = flat-sequence {
                    tunnel: [w239] -> w217
                    tunnel: [w237] -> w216
                    tunnel: [w249] -> w230
                    tunnel: [w250] -> w231
                    tunnel: [w242] -> w215
                    tunnel: [w246] -> _
                    tunnel: w229 -> [w243]
                    tunnel: w232 -> [w244]
                    frame #0 {
                      n124 = for {
                        N: "MFLI Averaging (Device2)" -> [_]
                        tunnel: [w264] -> w236 mode=indexing
                        tunnel: [w263] -> w238 mode=indexing
                        shift-right: [w266] -> w250
                        shift-left: w244 -> [w252]
                        shift-right: [w265] -> w249
                        shift-left: w243 -> [w251]
                        n125 = call-poly <instrlib>:"ziGetValue.vi"("error in"=w251, "Path"="demods/0/sample", "Handle In"=w252) -> ("error out"=w257:errorcluster, "Demod Sample Out"=w255:T3, "Handle Out"=w258:T2)
                        n126 = Unbundle By Name(w255) -> ("X (Vrms)"=w254:dbl, "Y (Vrms)"=w253:dbl)  [unwired: 1 out]
                        n127 = call-poly <instrlib>:"ziGetValue.vi"("error in"=w257, "Path"="demods/2/sample", "Handle In"=w258) -> ("error out"=w265:errorcluster, "Demod Sample Out"=w261:T3, "Handle Out"=w266:T2)
                        n128 = Unbundle By Name(w261) -> ("X (Vrms)"=w260:dbl, "Y (Vrms)"=w259:dbl)  [unwired: 1 out]
                        n129 = Re/Im To Polar(2:w253, 3:w254) -> (1:w263:dbl)  [unwired: 1 out]
                        n130 = Re/Im To Polar(2:w259, 3:w260) -> (1:w264:dbl)  [unwired: 1 out]
                      }
                      n131 = local read "Nanovoltmeter 2182a VISA (Device 2)"() -> (w246:refnum<visa-resource-name>)
                      n132 = for {
                        N: "DC Voltage averaging 2" -> [_]
                        tunnel: [w268] -> w247 mode=indexing
                        shift-right: [w267] -> _
                        shift-left: w246 -> [w269]
                        n133 = call "Get-V_K2182A_VISA_EL.vi"("VISA K2182A"=w269) -> ("V (V)"=w268:dbl, "VISA K2182A out"=w267:refnum<visa-resource-name>)  [unwired: 2 in, 1 out]
                      }
                      n134 = Add Array Elements(numeric array=w247) -> (sum=w248:dbl)
                      n135 = Divide(x=w248, y="DC Voltage averaging 2") -> (x/y=w242:dbl)
                      "DC Voltage (V) 2" <- w242
                      n136 = Add Array Elements(numeric array=w236) -> (sum=w240:dbl)
                      n137 = Add Array Elements(numeric array=w238) -> (sum=w241:dbl)
                      n138 = Divide(x=w240, y="MFLI Averaging (Device2)") -> (x/y=w237:dbl)
                      n139 = Divide(x=w241, y="MFLI Averaging (Device2)") -> (x/y=w239:dbl)
                    }
                  }
                  n140 = local read "Vset (V) 2"() -> (w224:dbl)
                  n141 = local read "Time (s)"() -> (w221:dbl)
                  n142 = Divide(x=w216, y=w217) -> (x/y=w219:dbl)
                  "dI/dV (ohm) 2" <- w219
                  n143 = Divide(x=w224, y="Resistance used for DC (ohm) 2") -> (x/y=w223:dbl)
                  n144 = Bundle(w215, w219) -> (w234:cluster{dbl, dbl})  [unwired: 1 in]
                  n145 = Build Array(w221, w215, w216, w217, w219, w224, w223) -> (w222:dbl[])
                  "data 2" <- w222
                  n146 = Build Array (concatenate)(w233, w234) -> (w218:cluster{dbl, "Field Reading":dbl}[])
                  "dI/dV vs DC Bias (Device 2)" <- w218
                  n147 = local read "File path 2"() -> (w226:path)
                  n148 = Array To Spreadsheet String(array=w222, 3:"%e" ("format string")) -> (spreadsheet string=w227:string)  [unwired: 1 in]
                  n149 = call <vilib>:"Write Characters To File.vi"("append to file? (new file:F)"=TRUE, "character string"=w227, "file path (dialog if empty)"=w226) -> ()  [unwired: 2 in, 1 out]
                  "dV (V) 2" <- w217
                  "dI (A) 2" <- w216
                }
              }
            }
          }
          n150 = call <instrlib>:"ziClose.vi"("Handle In"=w134) -> ()  [unwired: 1 in, 4 out]
          n151 = call <instrlib>:"ziClose.vi"("Handle In"=w127) -> ()  [unwired: 1 in, 4 out]
        }
      }
      n152 = Unbundle By Name(w115) -> ("status"=w114:bool)
      n153 = Or(x=w114, y="stop") -> ()  [unwired: 1 out]
    }
    frame #6 {
      w403 = 0.0
      w401 = 0
      w402 = 1
      n154 = call <instrlib>:"Configure Source (Level).vi"("VISA resource name"=w405, "Source Measure Unit Channel (0: Channel A)"=w401, "Level Type (1: Voltage)"=w402, "Voltage Level (0 V)"=w403) -> ("VISA resource name out"=w406:refnum<visa-resource-name>)  [unwired: 10 in, 1 out]
      n155 = call <instrlib>:"Enable Source Output.vi"("Output Mode (0: Turn off)"=w401, "Source Measure Unit Channel (0: Channel A)"=w401, "VISA resource name"=w406) -> ("VISA resource name out"=w400:refnum<visa-resource-name>)  [unwired: 7 in, 1 out]
      n156 = call <instrlib>:"Configure Source (Level).vi"("VISA resource name"=w400, "Source Measure Unit Channel (0: Channel A)"=w402, "Level Type (1: Voltage)"=w402, "Voltage Level (0 V)"=w403) -> ("VISA resource name out"=w404:refnum<visa-resource-name>)  [unwired: 10 in, 1 out]
      n157 = call <instrlib>:"Enable Source Output.vi"("Output Mode (0: Turn off)"=w401, "Source Measure Unit Channel (0: Channel A)"=w402, "VISA resource name"=w404) -> ("VISA resource name out"=w399:refnum<visa-resource-name>)  [unwired: 7 in, 1 out]
      n158 = call <instrlib>:"Close.vi"("VISA resource name"=w399) -> ()  [unwired: 10 in, 1 out]
    }
  }
